vi "route.vi"() -> ()   [LabVIEW 2014]
uses:
  <vilib>/Utility/sysdir.llb/System Directory Type.ctl
  <vilib>/Utility/config.llb/Read Key (String).vi
  <vilib>/Utility/config.llb/Write Key (String).vi
  <vilib>/Utility/config.llb/Read Key (Path).vi
  <vilib>/Utility/config.llb/Write Key (Path).vi
  subVI/departure.vi
  subVI/Destination.vi
  <vilib>/Utility/file.llb/Write To Spreadsheet File (string).vi
  <vilib>/httpClient/LabVIEWHTTPClient.lvlib
  <vilib>/Utility/config.llb/NI_LVConfig.lvlib
panel:
  in  "?":bool
  in  "?":bool
  in  "?":bool
  out "PMDG":string
  out "FS2004/FS9":string
  out "FSX":string
  out "활주로 2":string[](array[string])
  out "초":i32[](array[numeric])
  out "분":i32[](array[numeric])
  out "시":i32[](array[numeric])
  in  "기록":bool
  out "시간 2":string
  in  "확인 버튼 2":bool
  in  "초기화 2":bool
  out "시간":string
  in  "ATC":bool
  out "활주로":string[](array[string])
  out "fms":string
  out "time/시간":dbl
  in  "도움말":bool
  in  "피드백":bool
  in  "저장 경로":path
  out "Distance":string="0"
  in  "찾기":bool
  in  "?":bool
  in  "?":bool
  out "x fmc 플랜":string
  out "FMS 플랜":string
  in  "Destination":string
  in  "departure":string
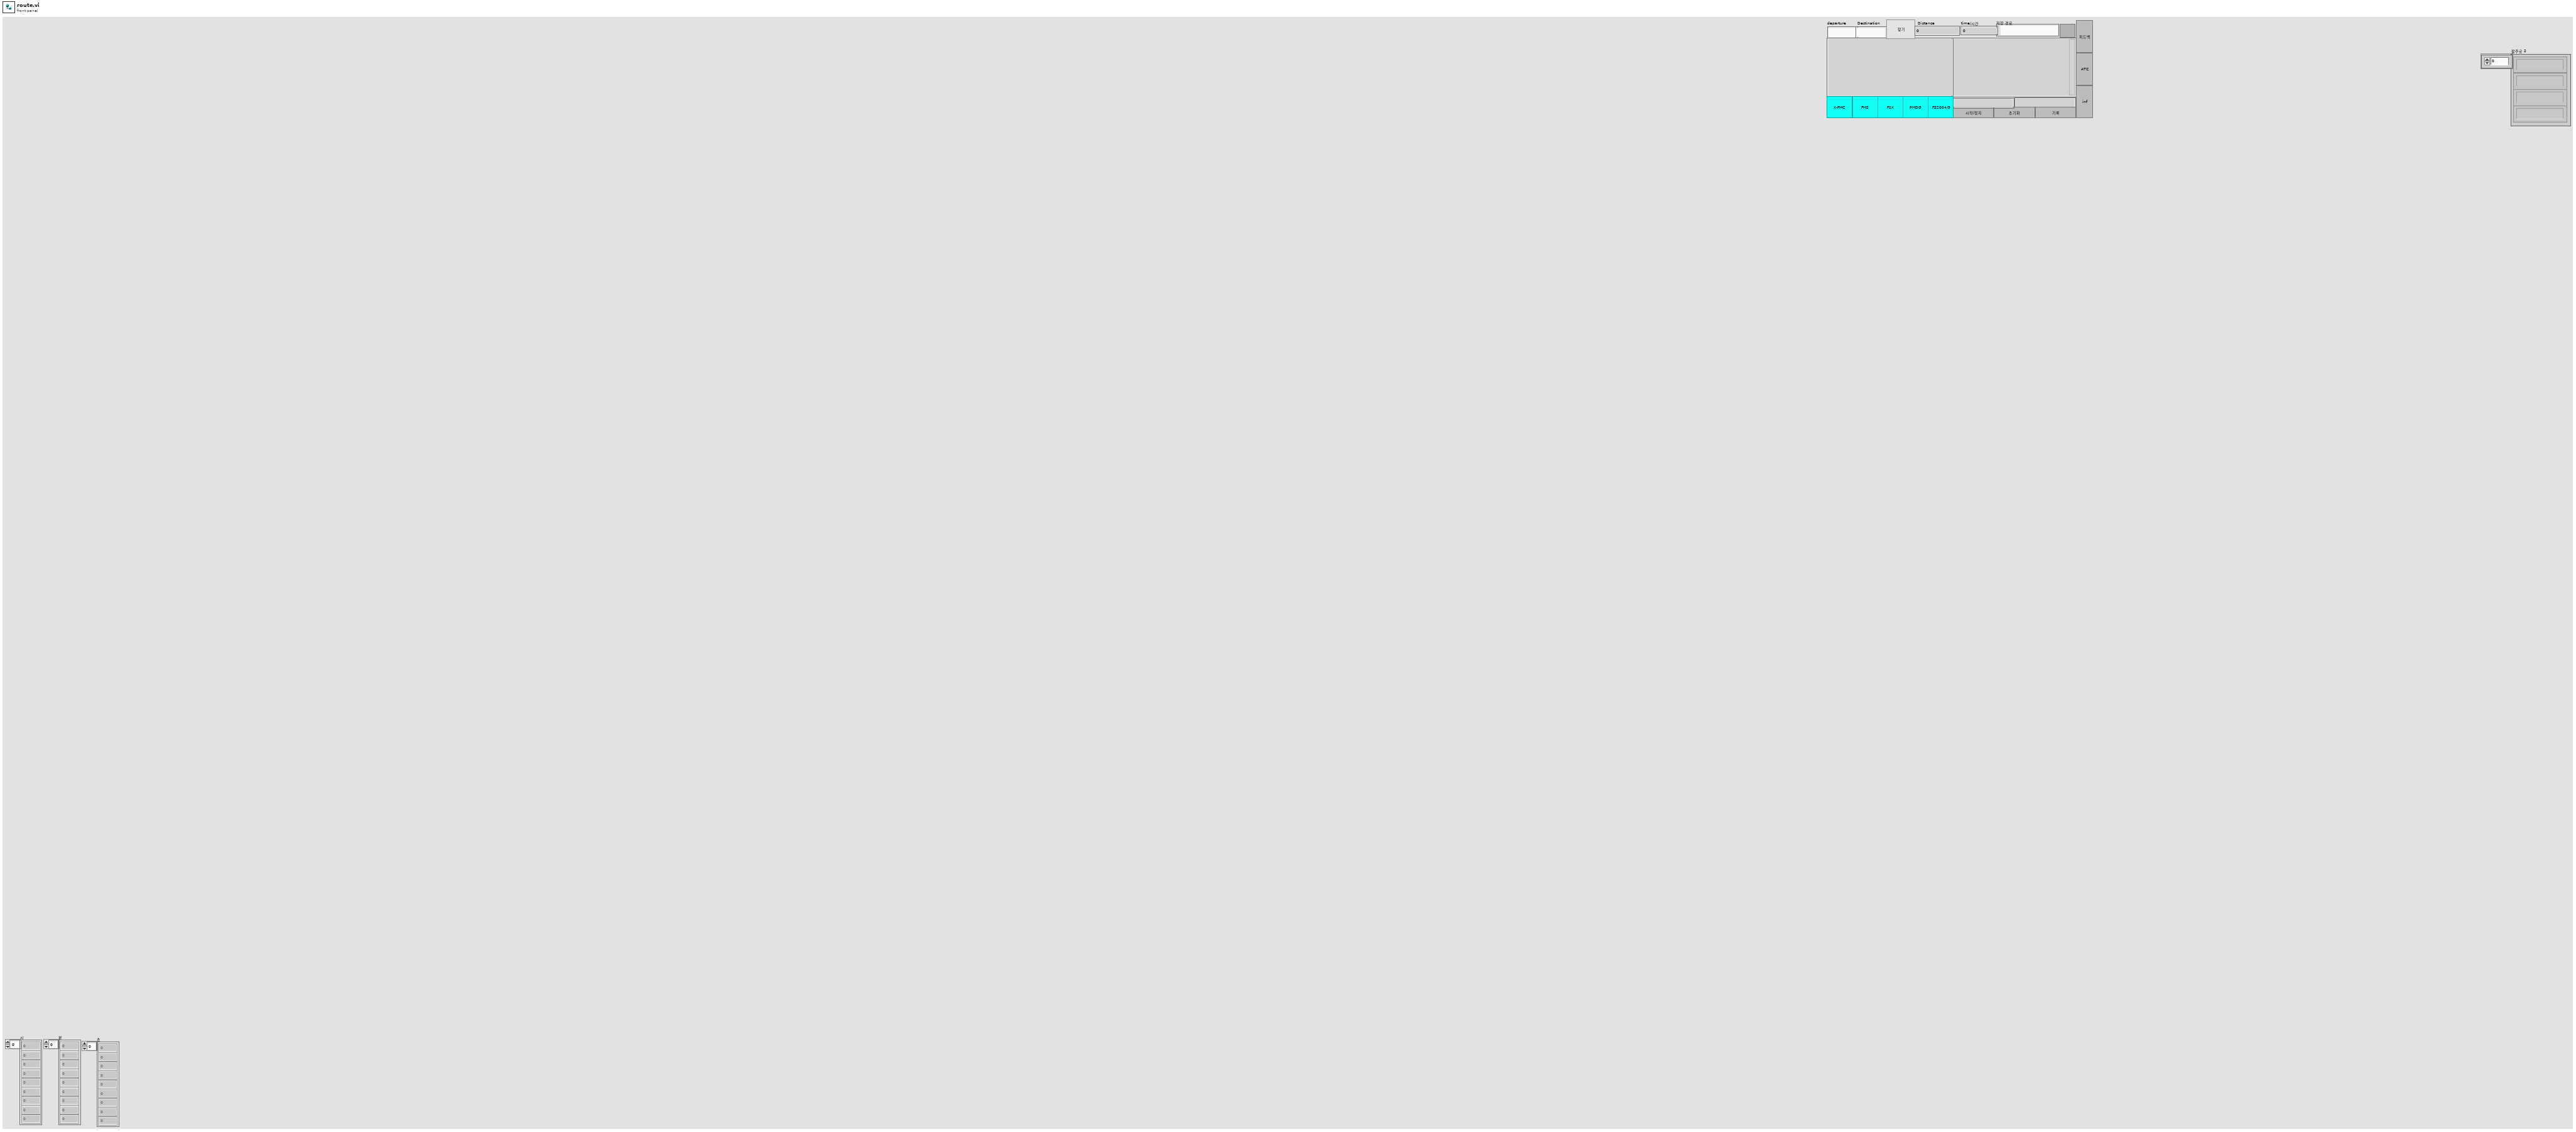
[diagram p1: front panel]
types:
  T1 = enum16{"open", "replace", "create", "open or create", "replace or create", "replace or create with confirmation"}
  T2 = typedef "NI_LVConfig.lvlib/Config Data RefNum.ctl" = refnum<k1>
  T3 = typedef "System Directory Type.ctl" = i32
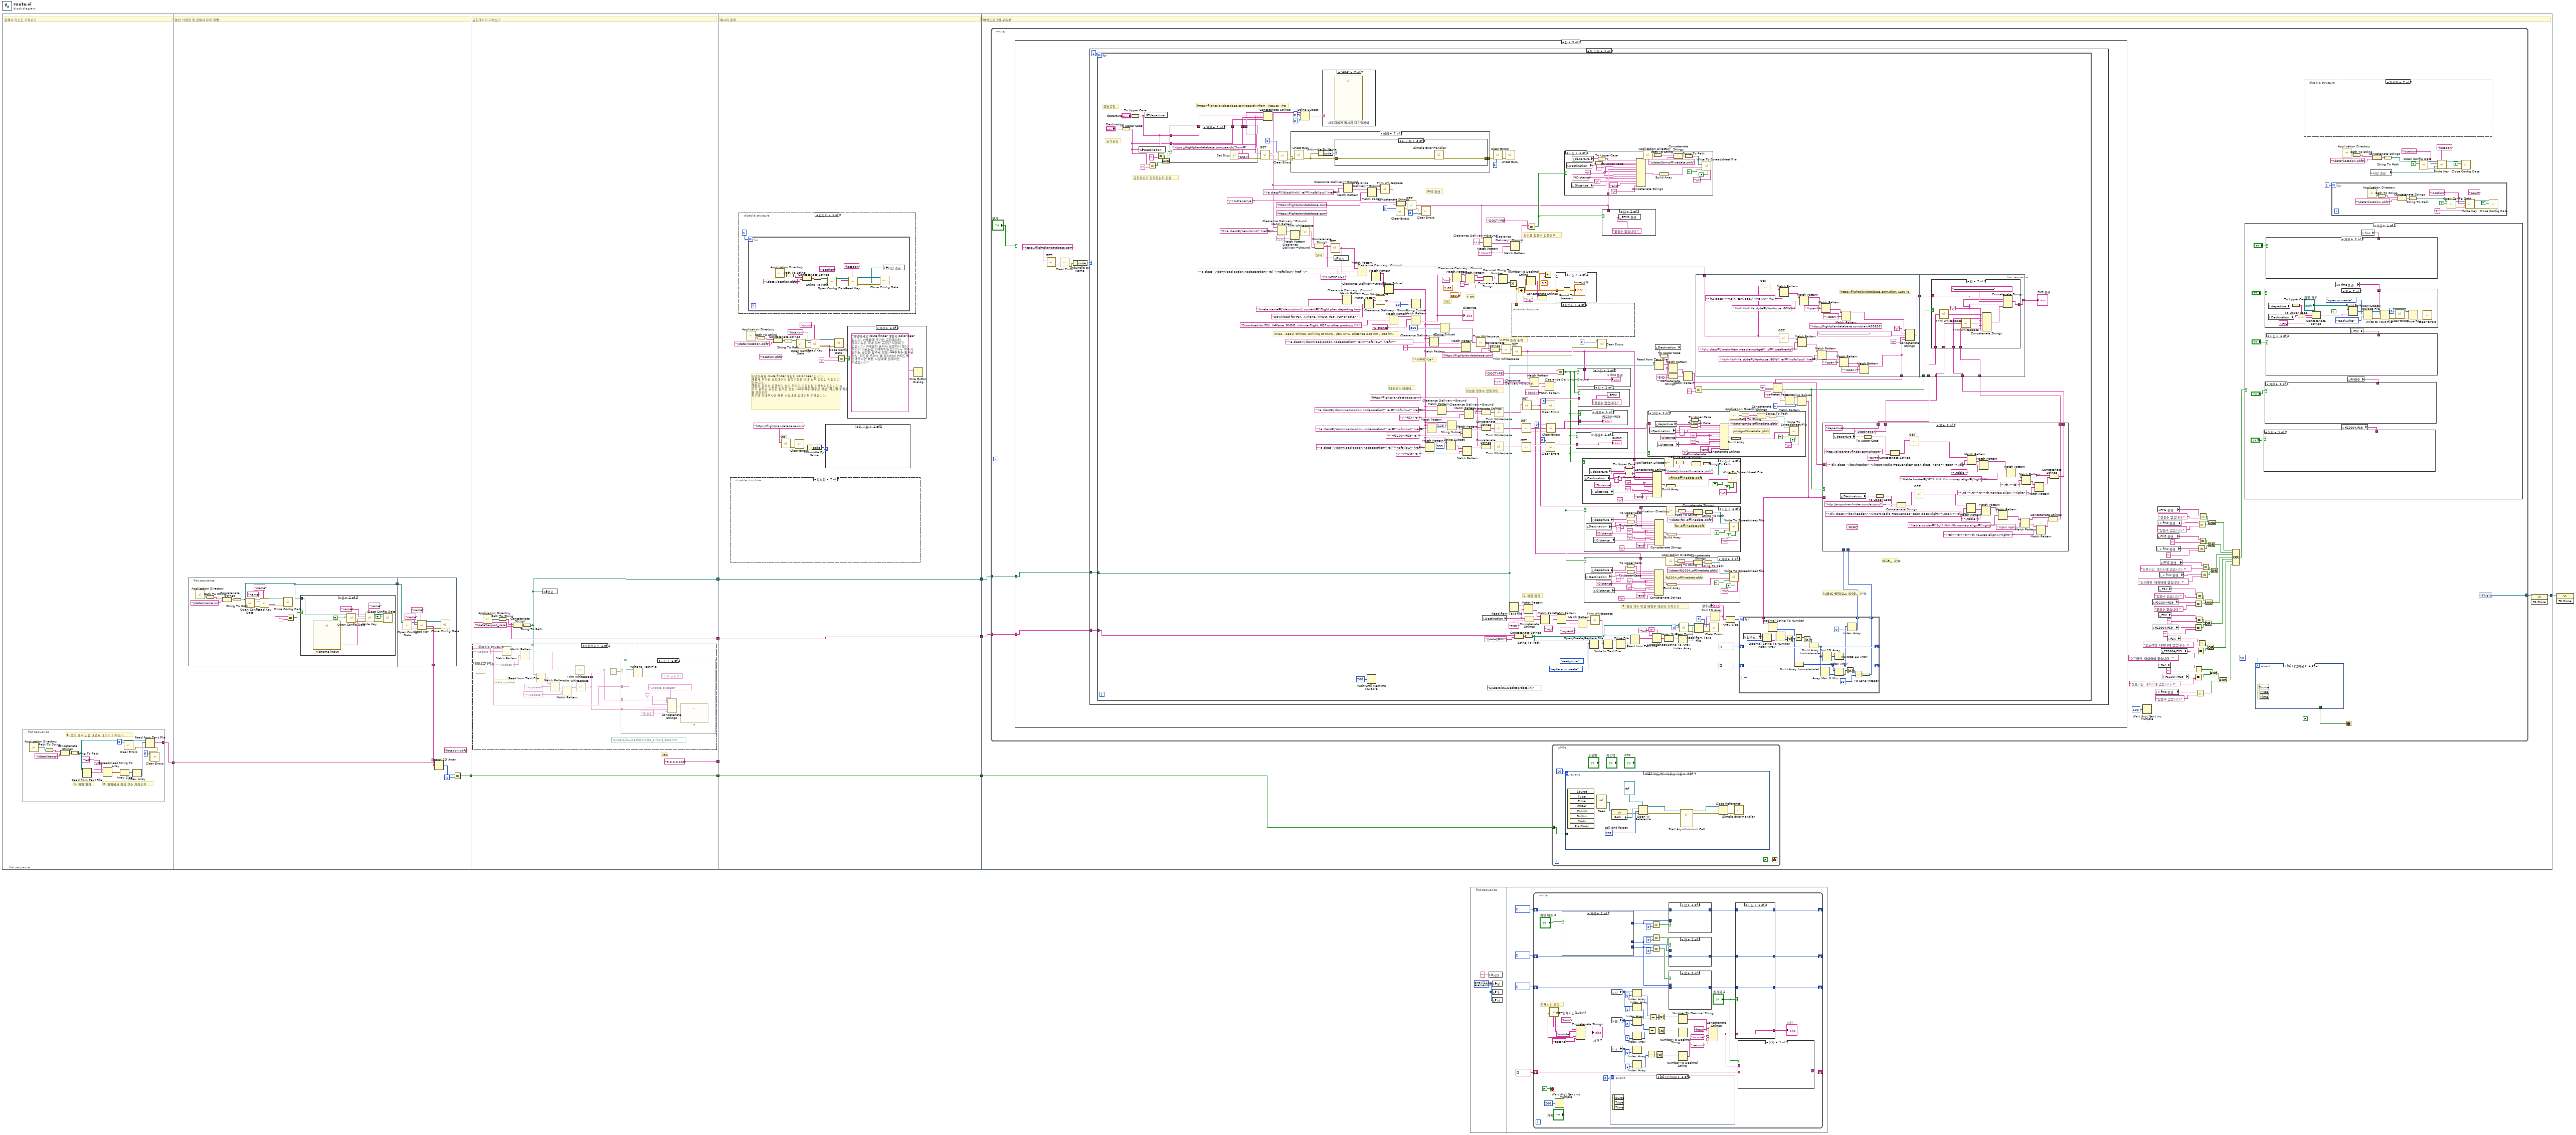
[diagram p0: block diagram]
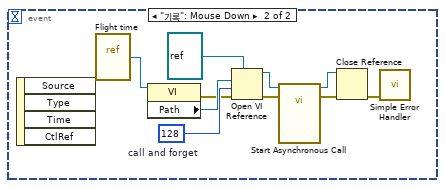
[diagram p2: hidden frame]
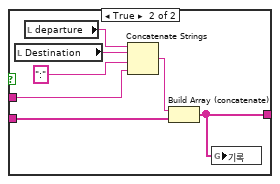
[diagram p3: hidden frame]
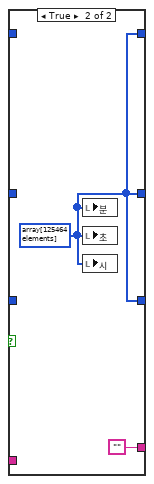
[diagram p4: hidden frame]
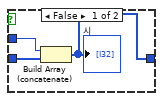
[diagram p5: hidden frame]
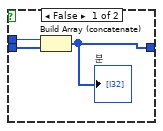
[diagram p6: hidden frame]
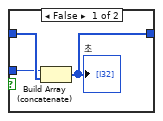
[diagram p7: hidden frame]
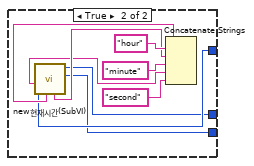
[diagram p8: hidden frame]
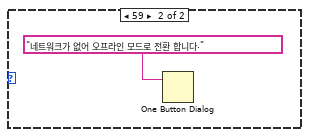
[diagram p13: hidden frame]
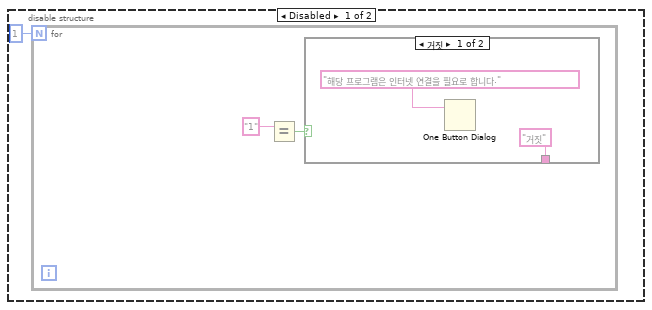
[diagram p14: hidden frame]
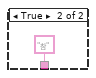
[diagram p15: hidden frame]
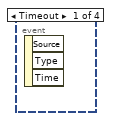
[diagram p17: hidden frame]
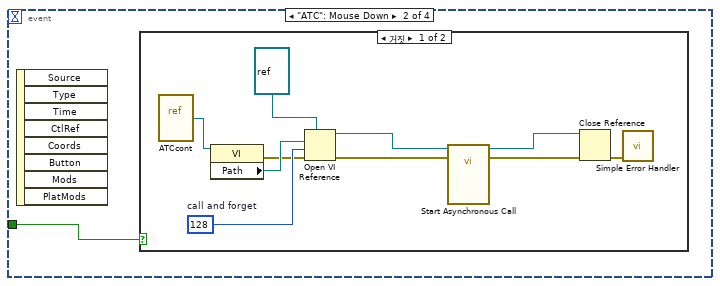
[diagram p18: hidden frame]
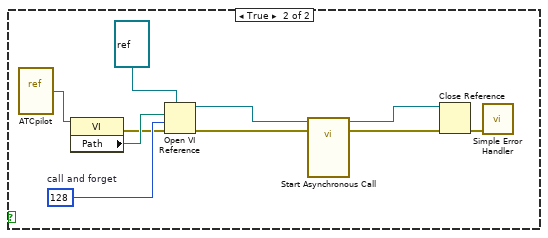
[diagram p19: hidden frame]
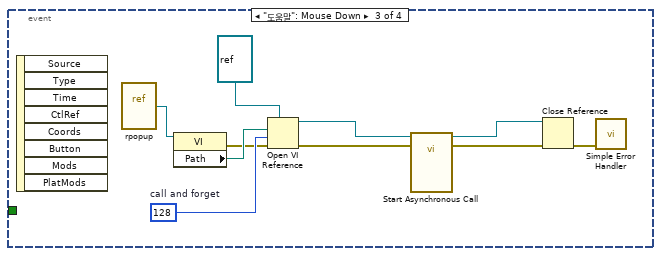
[diagram p20: hidden frame]
diagram:
  n1 = flat-sequence {
    tunnel: [w11] -> w5
    tunnel: w5 -> [w33]
    tunnel: [w31] -> w4
    tunnel: [w69] -> w8
    tunnel: [w70] -> w7
    tunnel: ["3.0.0.0.100"] -> w6
    tunnel: w4 -> [w66]
    tunnel: [w66] -> w3
    tunnel: [w97] -> w10
    tunnel: [w98] -> w9
    tunnel: w8 -> [w97]
    tunnel: w7 -> [w98]
    tunnel: w6 -> [_]
    tunnel: w3 -> [w96]
    tunnel: [w96] -> w2
    tunnel: w10 -> [w142]
    tunnel: w9 -> [w141]
    tunnel: w2 -> [w140]
    tunnel: [w138] -> w1
    frame #0 {
      # "관제사 리스드 가져오기"
      n2 = flat-sequence {
        tunnel: [w16] -> w11
        frame #0 {
          # "3. 행의 갯수 만큼 배열로 데이터 가져오기"
          # "2. 파일에서 행의 갯수 가져오기"
          # "1. 파일 읽기"
          n3 = call <vilib>:"Application Directory.vi"() -> ("Application Directory"=w20:path)
          n4 = Path To String(path=w20) -> (string=w19:string)
          n5 = Concatenate Strings(w19, "\\data\\temp" ("문자열")) -> (w18:string)
          n6 = String To Path(string=w18) -> (path=w17:path)
          n7 = Read from Text File(file (use dialog)=w17) -> (text=w23:string)  [unwired: 1 in, 5 out]
          n8 = Spreadsheet String To Array(delimiter (Tab)="\r", format string="%d", spreadsheet string=w23) -> (array=w25:dbl[][])  [unwired: 1 out]
          n9 = Array Size(array=w25) -> (size(s)=w24:i32[])
          n10 = call <vilib>:"Clear Errors.vi"("specific error code to clear (0: all)"=0) -> ("error out"=w15:errorcluster)  [unwired: 5 in, 1 out]
          n11 = Index Array(array=w24) -> (element=w22:i32)  [unwired: 1 in]
          n12 = Read from Text File(file (use dialog)=w17, count=w22, error in=w15) -> (text=w16:string[], error out=w13:errorcluster)  [unwired: 3 out]
          n13 = call <vilib>:"Clear Errors.vi"("error in (no error)"=w13, "specific error code to clear (0: all)"=0) -> ()  [unwired: 4 in, 2 out]
        }
      }
    }
    frame #1 {
      (unwired) "location.pbfs" ("문자열")
      # "본인 닉네임 및 관제사 유무 판별"
      n14 = flat-sequence {
        tunnel: [w34] -> w28
        tunnel: [w59] -> w30
        tunnel: w28 -> [w58]
        frame #0 {
          n15 = call <vilib>:"Application Directory.vi"() -> ("Application Directory"=w40:path)
          n16 = Path To String(path=w40) -> (string=w38:string)
          n17 = Concatenate Strings(w38, "\\data\\name.ini" ("문자열")) -> (w39:string)
          n18 = String To Path(string=w39) -> (path=w34:path)
          n19 = call <vilib>:"Open Config Data.vi"("configuration file path"=w34) -> ("error out"=w45:errorcluster, "refnum"=w46:T2)  [unwired: 8 in, 1 out]
          n20 = call-poly <vilib>:"Read Key.vi"("section"="name", "error in (no error)"=w45, "key"="name", "refnum"=w46) -> ("error out"=w44:errorcluster, "value"=w35:string, "refnum out"=w43:T2)  [unwired: 4 in, 1 out]
          n21 = call <vilib>:"Close Config Data.vi"("error in (no error)"=w44, "refnum"=w43) -> ()  [unwired: 8 in, 2 out]
          n22 = Equal?(x=w35, y="") -> (x = y?=w36:bool)
          n23 = case shown="참" w36 {
            tunnel: w34 -> [_ w48]
            frame False {
            }
            frame True {
              n24 = call "nicname input"() -> ("nicname"=w49:string)  [unwired: 17 in, 2 out]
              n25 = call <vilib>:"Open Config Data.vi"("create file if necessary (T)"=TRUE, "configuration file path"=w48) -> ("error out"=w51:errorcluster, "refnum"=w52:T2)  [unwired: 7 in, 1 out]
              n26 = call-poly <vilib>:"Write Key.vi"("section"="name", "error in (no error)"=w51, "value"=w49, "key"="name", "refnum"=w52) -> ("error out"=w54:errorcluster, "refnum out"=w53:T2)  [unwired: 4 in, 1 out]
              n27 = call <vilib>:"Close Config Data.vi"("error in (no error)"=w54, "write file if changed (T)"=TRUE, "refnum"=w53) -> ()  [unwired: 7 in, 2 out]
            }
          }
        }
        frame #1 {
          n28 = call <vilib>:"Open Config Data.vi"("configuration file path"=w58) -> ("error out"=w62:errorcluster, "refnum"=w61:T2)  [unwired: 8 in, 1 out]
          n29 = call-poly <vilib>:"Read Key.vi"("section"="name", "error in (no error)"=w62, "key"="name", "refnum"=w61) -> ("error out"=w63:errorcluster, "value"=w59:string, "refnum out"=w64:T2)  [unwired: 4 in, 1 out]
          n30 = call <vilib>:"Close Config Data.vi"("error in (no error)"=w63, "refnum"=w64) -> ()  [unwired: 8 in, 2 out]
        }
      }
      n31 = Search 1D Array(1D array=w33, element=w30) -> (index of element=w32:i32)  [unwired: 1 in]
      n32 = Equal?(x=w32, y=-1) -> (x = y?=w31:bool)
    }
    frame #2 {
      # "VER"
      # "공항데이터 가져오기"
      n33 = call <vilib>:"Application Directory.vi"() -> ("Application Directory"=w72:path)
      n34 = Path To String(path=w72) -> (string=w70:string)
      n35 = Concatenate Strings(w70, "\\data\\airport_data" ("문자열")) -> (w68:string)
      n36 = String To Path(string=w68) -> (path=w69:path)
      n37 = disable-structure shown="비활성화" {
        disable-tunnel: w69 -> [w86 _]
        frame Disabled {
          (unwired) path "C:/Users/lsw/Desktop/KOR_airport_data.txt" ("File Path Control")
          # "data update"
          n38 = call "데이터업데이트.vi"() -> ("data"=w76:string)  [unwired: 11 in]
          n39 = Match Pattern(string=w76, regular expression="<update>" ("정규식")) -> (after substring=w84:string)  [unwired: 1 in, 3 out]
          n40 = Match Pattern(string=w84, regular expression="</update>" ("정규식")) -> (before substring=w78:string)  [unwired: 1 in, 3 out]
          n41 = Read from Text File(file (use dialog)=w86) -> (text=w79:string)  [unwired: 3 in, 3 out]
          n42 = Match Pattern(string=w79, regular expression="<update>" ("정규식")) -> (after substring=w81:string)  [unwired: 1 in, 3 out]
          n43 = Match Pattern(string=w81, regular expression="</update>" ("정규식")) -> (before substring=w77:string)  [unwired: 1 in, 3 out]
          n44 = call <vilib>:"Trim Whitespace.vi"("string"=w78) -> ("trimmed string"=w74:string)  [unwired: 1 in]
          n45 = call <vilib>:"Trim Whitespace.vi"("string"=w77) -> ("trimmed string"=w75:string)  [unwired: 1 in]
          n46 = Equal?(x=w74, y=w75) -> (x = y?=w73:bool)
          n47 = case shown="거짓" w73 {
            tunnel: w86 -> [w95 _]
            tunnel: w76 -> [w89 _]
            tunnel: w75 -> [w88 _]
            tunnel: w74 -> [w87 _]
            frame False {
              n48 = Write to Text File(file (use dialog)=w95, text=w89) -> ()  [unwired: 2 in, 3 out]
              n49 = Concatenate Strings(w87, "update success" ("문자열"), "\r", "기존 버전은", w88, "입니다." ("문자열")) -> (w90:string)
              n50 = call "?"("Message"=w90) -> ()  [unwired: 9 in, 2 out]
            }
            frame True {
            }
          }
        }
        frame Enabled {
        }
      }
      n51 = global write "airport경로.vi" "경로"(w69) -> ()
    }
    frame #3 {
      (unwired) "location.pbfs" ("문자열")
      # "안녕하세요 route finder 개발자 polor bear 입니다. \n새롭게 추가된 공항데이터 출력기능은 국내 일부 공항만 지원되고 있습니다. \n개발자 혼자서 진행하다 보니 무리가 따르는점 이해부탁드립니다.ㅠ \n추가 원하는 공항은 활주로 정보,.ILS주파수,활주로 정보  파드별 주파수 를 정리하여 \n피드백 보내주시면 빠른 시일내에 업데이트 하겟습니다."
      # "메시지 출력"
      n52 = disable-structure shown="활성화" {
        frame Disabled {
          n53 = for {
            N: 1 -> [_]
            n54 = Equal?(x="1" ("y")) -> (x = y?=w121:bool)  [unwired: 1 in]
            n55 = case shown="거짓" w121 {
              tunnel: ["거짓" "참"] -> _
              frame False {
                n56 = One Button Dialog(message="해당 프로그램은 인터넷 연결을 필요로 합니다." ("메시지")) -> ()  [unwired: 1 in, 1 out]
              }
              frame True {
              }
            }
          }
        }
        frame Enabled {
        }
      }
      n57 = disable-structure shown="활성화" {
        frame Enabled {
          n58 = for {
            N: 1 -> [_]
            n59 = call <vilib>:"Application Directory.vi"() -> ("Application Directory"=w129:path)
            n60 = Path To String(path=w129) -> (string=w127:string)
            n61 = Concatenate Strings(w127, "\\data\\location.pbfs" ("문자열")) -> (w128:string)
            n62 = String To Path(string=w128) -> (path=w126:path)
            n63 = call <vilib>:"Open Config Data.vi"("configuration file path"=w126) -> ("error out"=w135:errorcluster, "refnum"=w134:T2)  [unwired: 8 in, 1 out]
            n64 = call-poly <vilib>:"Read Key.vi"("section"="location", "error in (no error)"=w135, "key"="location", "refnum"=w134) -> ("error out"=w136:errorcluster, "value"=w131:path, "refnum out"=w137:T2)  [unwired: 4 in, 1 out]
            n65 = call <vilib>:"Close Config Data.vi"("error in (no error)"=w136, "refnum"=w137) -> ()  [unwired: 8 in, 2 out]
            n66 = local write "저장 경로"(w131) -> ()
          }
        }
        frame Disabled {
        }
      }
      n67 = call <vilib>:"Application Directory.vi"() -> ("Application Directory"=w102:path)
      n68 = Path To String(path=w102) -> (string=w100:string)
      n69 = Concatenate Strings(w100, "\\data\\location.pbfs" ("문자열")) -> (w101:string)
      n70 = call <vilib>:"GET.vi"("url"="https://flightplandatabase.com") -> ("error out"=w116:errorcluster)  [unwired: 11 in, 3 out]
      n71 = String To Path(string=w101) -> (path=w99:path)
      n72 = call <vilib>:"Clear Errors.vi"("error in (no error)"=w116) -> ("error out"=w114:errorcluster)  [unwired: 5 in, 1 out]
      n73 = call <vilib>:"Open Config Data.vi"("configuration file path"=w99) -> ("error out"=w110:errorcluster, "refnum"=w111:T2)  [unwired: 8 in, 1 out]
      n74 = Unbundle By Name(w114) -> ("code"=w113:i32)
      n75 = call-poly <vilib>:"Read Key.vi"("section"="count", "error in (no error)"=w110, "key"="location", "refnum"=w111) -> ("error out"=w109:errorcluster, "value"=w104:string, "refnum out"=w108:T2)  [unwired: 4 in, 1 out]
      n76 = case shown="0, 기본" w113 {
        frame 0, Default {
        }
        frame 59 {
          n77 = One Button Dialog(message="네트워크가 없어 오프라인 모드로 전환 합니다." ("메시지")) -> ()  [unwired: 1 in, 1 out]
        }
      }
      n78 = call <vilib>:"Close Config Data.vi"("error in (no error)"=w109, "refnum"=w108) -> ()  [unwired: 8 in, 2 out]
      n79 = Equal?(x=w104, y="1") -> (x = y?=w106:bool)
      n80 = case shown="거짓" w106 {
        frame False {
          n81 = One Button Dialog(message="안녕하세요 route finder 개발자 polor bear 입니다. \n새롭게 추가된 공항데이터 출력기능은 국내 일부 공항만 지원되고 있습니다. \n개발자 혼자서 진행하다 보니 무리가 따르는점 이해부탁드립니다.ㅠ \n추가 원하는 공항은 활주로 정보,.ILS주파수,활주로 정보  파드별 주파수 를 정리하여 \n피드백 보내주시면 빠른 시일내에 업데이트 하겟습니다." ("메시지")) -> ()  [unwired: 1 in, 1 out]
        }
        frame True {
        }
      }
    }
    frame #4 {
      # "메인프로그램 구동부"
      n82 = while {
        tunnel: w142 -> [w231]
        tunnel: w141 -> [w230]
        tunnel: [w220] -> w139
        stop <- w221 stop-if-true
        (unwired) FALSE
        n83 = case shown="참" "찾기" {
          tunnel: w231 -> [w280 w526]
          tunnel: w230 -> [w279 w525]
          frame False {
            n84 = disable-structure shown="비활성화" {
              disable-tunnel: w280 -> [w282 _]
              disable-tunnel: w279 -> [w281 _]
              frame Disabled {
                n85 = while {
                  tunnel: w282 -> [w297]
                  tunnel: w281 -> [w296]
                  stop <- FALSE stop-if-true
                  (unwired) path "C:/Users/lsw/Desktop/data.ini" ("File Path Control")
                  # "¼Œ·tÇ ÆÅDÇLµ \\ÖüÈ\\¸  ÁÝÐ"
                  # "1. 파일 읽기"
                  # "3. 행의 갯수 만큼 배열로 데이터 가져오기"
                  n86 = local read "Destination"() -> (w284:string)
                  n87 = Wait Until Next ms Multiple(millisecond multiple=u32 1800000 ("ms 배수")) -> ()  [unwired: 1 out]
                  n88 = Equal?(x="", y=w284) -> (x = y?=w285:bool)
                  n89 = case shown="참" w285 {
                    tunnel: w284 -> [_ w355]
                    tunnel: [_ w354] -> w286
                    frame False {
                    }
                    frame True {
                      n90 = To Upper Case(1:w355) -> (0:w354:string)
                    }
                  }
                  n91 = local read "Destination"() -> (w288:string)
                  n92 = Concatenate Strings(w296, "\\data\\RWY" ("문자열")) -> (w350:string)
                  n93 = Read from Text File(file (use dialog)=w297) -> (text=w337:string)  [unwired: 1 in, 5 out]
                  n94 = String To Path(string=w350) -> (path=w352:path)
                  n95 = Equal?(x=w288, y="") -> (x = y?=w289:bool)
                  n96 = Match Pattern(string=w337, regular expression=w286) -> (after substring=w336:string)  [unwired: 1 in, 3 out]
                  n97 = Concatenate Strings(w286, "END;" ("정규식")) -> (w339:string)
                  n98 = case shown="거짓" w289 {
                    tunnel: w288 -> [w356 _]
                    tunnel: [w356 _] -> w290
                    frame False {
                    }
                    frame True {
                    }
                  }
                  n99 = Match Pattern(string=w336, regular expression=w339) -> (before substring=w338:string)  [unwired: 1 in, 3 out]
                  n100 = Match Pattern(string=w338, regular expression="rwy" ("문자열")) -> (after substring=w341:string)  [unwired: 1 in, 3 out]
                  n101 = Read from Text File(file (use dialog)=w297) -> (text=w312:string)  [unwired: 1 in, 5 out]
                  n102 = To Upper Case(1:w290) -> (0:w317:string)
                  n103 = Match Pattern(string=w341, regular expression="rwyand;" ("정규식")) -> (before substring=w342:string)  [unwired: 1 in, 3 out]
                  n104 = Concatenate Strings(w317, "END;" ("정규식")) -> (w314:string)
                  n105 = Match Pattern(string=w312, regular expression=w317) -> (after substring=w316:string)  [unwired: 1 in, 3 out]
                  n106 = call <vilib>:"Trim Whitespace.vi"("string"=w342) -> ("trimmed string"=w343:string)  [unwired: 1 in]
                  n107 = Match Pattern(string=w316, regular expression=w314) -> (before substring=w299:string)  [unwired: 1 in, 3 out]
                  n108 = Open/Create/Replace File(file path (use dialog)=w352, operation (0:open)=T1."replace or create" ("동작(0:open)"), access (0:read/write)=enum16{"read/write", "read-only", "write-only"}."read/write" ("접근(0:읽기/쓰기)")) -> (refnum out=w347:refnum<file>, error out=w344:errorcluster)  [unwired: 3 in, 1 out]
                  n109 = Write to Text File(file (use dialog)=w347, text=w343, error in=w344) -> (refnum out=w346:refnum<file>, error out=w345:errorcluster)  [unwired: 1 in, 1 out]
                  n110 = Equal?(x=w299, y="") -> (x = y?=w298:bool)
                  n111 = Close File(refnum=w346, error in=w345) -> (error out=w318:errorcluster)  [unwired: 1 out]
                  n112 = global read "날시.vi" "날시"() -> (w294:string)
                  n113 = Read from Text File(file (use dialog)=w352, error in=w318) -> (text=w324:string)  [unwired: 5 out]
                  n114 = Spreadsheet String To Array(delimiter (Tab)="\r", format string="%d", spreadsheet string=w324) -> (array=w326:dbl[][])  [unwired: 1 out]
                  n115 = flat-sequence {
                    tunnel: w294 -> [w359]
                    tunnel: [w358] -> w353
                    tunnel: [w357] -> w295
                    tunnel: w301 -> [w386]
                    tunnel: w300 -> [w384]
                    tunnel: w353 -> [w385]
                    tunnel: w303 -> [w383]
                    tunnel: w302 -> [w381]
                    tunnel: [w382] -> w293
                    tunnel: [w380] -> _
                    tunnel: w298 -> [w380]
                    frame #0 {
                      (unwired) "https://flightplandatabase.com/plan/435659"
                      # "https://flightplandatabase.com/plan/425078"
                      n116 = call <vilib>:"GET.vi"("url"=w359) -> ("body"=w379:string)  [unwired: 11 in, 3 out]
                      n117 = call <vilib>:"GET.vi"("url"=w359) -> ("body"=w364:string)  [unwired: 11 in, 3 out]
                      n118 = Match Pattern(string=w379, regular expression="<h2 class=\"main-item-title\">METAR</h2>" ("정규식")) -> (after substring=w377:string)  [unwired: 1 in, 3 out]
                      n119 = Match Pattern(string=w364, regular expression="<div class=\"main-item weather-widget\" id=\"weather-to\">" ("정규식")) -> (after substring=w366:string)  [unwired: 1 in, 3 out]
                      n120 = Match Pattern(string=w377, regular expression="<br><br><a style=\"font-size: 80%\" " ("정규식")) -> (before substring=w375:string)  [unwired: 1 in, 3 out]
                      n121 = Match Pattern(string=w366, regular expression="<br><br><a style=\"font-size: 80%\" rel=\"nofollow\" href=\"" ("정규식")) -> (before substring=w368:string)  [unwired: 1 in, 3 out]
                      n122 = Match Pattern(string=w375, regular expression="<span>" ("정규식")) -> (after substring=w373:string)  [unwired: 1 in, 3 out]
                      n123 = Match Pattern(string=w368, regular expression="<span>" ("정규식")) -> (after substring=w370:string)  [unwired: 1 in, 3 out]
                      n124 = Match Pattern(string=w373, regular expression="</span>" ("정규식")) -> (before substring=w361:string)  [unwired: 1 in, 3 out]
                      n125 = Match Pattern(string=w370, regular expression="</span>" ("정규식")) -> (before substring=w357:string)  [unwired: 1 in, 3 out]
                      n126 = Concatenate Strings(w361, "\r", "-------------------------------------------------" ("문자열"), "\r", w357) -> (w358:string)
                    }
                    frame #1 {
                      n127 = case shown="참" w380 {
                        tunnel: w386 -> [w394 w404]
                        tunnel: w385 -> [w395 w403]
                        tunnel: w384 -> [w387 w402]
                        tunnel: w383 -> [_ w400]
                        tunnel: w381 -> [w390 w398]
                        tunnel: [w393 w397] -> w382
                        frame False {
                          w389 = "\r"
                          n128 = call <vilib>:"Trim Whitespace.vi"("string"=w387) -> ("trimmed string"=w388:string)  [unwired: 1 in]
                          n129 = Concatenate Strings(w390, w389, w389, w394, w389, w388) -> (w391:string)
                          n130 = call <vilib>:"Trim Whitespace.vi"("string"=w391) -> ("trimmed string"=w392:string)  [unwired: 1 in]
                          n131 = Concatenate Strings(w395, w389, "--------------frequency------------" ("문자열"), w389, w392) -> (w393:string)
                        }
                        frame True {
                          w405 = "\r"
                          n132 = call <vilib>:"Trim Whitespace.vi"("string"=w400) -> ("trimmed string"=w401:string)  [unwired: 1 in]
                          n133 = call <vilib>:"Trim Whitespace.vi"("string"=w398) -> ("trimmed string"=w399:string)  [unwired: 1 in]
                          n134 = Concatenate Strings(w401, w405, w404, w405, w399, w405, w402, w405) -> (w406:string)
                          n135 = Concatenate Strings(w403, w405, "----------------------------------------" ("문자열"), w405, w406) -> (w397:string)
                        }
                      }
                    }
                  }
                  n136 = Array Size(array=w326) -> (size(s)=w325:i32[])
                  n137 = Index Array(array=w325) -> (element=w323:i32)  [unwired: 1 in]
                  n138 = call <vilib>:"Clear Errors.vi"("specific error code to clear (0: all)"=0) -> ("error out"=w329:errorcluster)  [unwired: 5 in, 1 out]
                  n139 = Read from Text File(file (use dialog)=w352, count=w323, error in=w329) -> (text=w333:string[], error out=w331:errorcluster)  [unwired: 3 out]
                  n140 = call <vilib>:"Clear Errors.vi"("error in (no error)"=w331, "specific error code to clear (0: all)"=0) -> ()  [unwired: 4 in, 2 out]
                  n141 = Match Pattern(string=w295, regular expression="Z" ("정규식")) -> (after substring=w308:string)  [unwired: 1 in, 3 out]
                  n142 = Sort 1D Array(array=w333) -> (sorted array=w319:string[])
                  "활주로 2" <- w319
                  n143 = Match Pattern(string=w308, regular expression="KT" ("정규식")) -> (before substring=w310:string)  [unwired: 1 in, 3 out]
                  n144 = Array Size(array=w319) -> (size(s)=w321:i32)
                  n145 = String Subset(string=w310, length (rest)=4 ("길이(나머지)")) -> (substring=w306:string)  [unwired: 1 in]
                  n146 = for {
                    N: w321 -> [_]
                    shift-right: [w519] -> _
                    shift-left: i32[] [] -> [w523]
                    shift-right: [w505] -> _
                    shift-left: i32[] [] -> [w517]
                    tunnel: w306 -> [w509]
                    tunnel: [w506] -> w304 mode=indexing
                    tunnel: [w503] -> w305 mode=indexing
                    i -> [w524]
                    n147 = local read "활주로 2"() -> (w522:string[])
                    n148 = Index Array(array=w522, index=w524) -> (element=w521:string)
                    n149 = Decimal String To Number(string=w521) -> (number=w513:i32)  [unwired: 2 in, 1 out]
                    n150 = Decimal String To Number(string=w509) -> (number=w508:i32)  [unwired: 2 in, 1 out]
                    n151 = Absolute Value(x=w513) -> (abs(x)=w507:i32)
                    n152 = Subtract(x=w508, y=w507) -> (x-y=w512:i32)
                    n153 = Build Array (concatenate)(w507, w517) -> (w505:i32[])
                    n154 = Absolute Value(x=w512) -> (abs(x)=w511:i32)
                    n155 = Build Array (concatenate)(w511, w523) -> (w519:i32[])
                    n156 = Array Max & Min(array=w519) -> (min index (indices)=w518:i32)  [unwired: 3 out]
                    n157 = Sort 1D Array(array=w519) -> (sorted array=w520:i32[])
                    n158 = Reverse 1D Array(array=w520) -> ()  [unwired: 1 out]
                    n159 = Index Array(array=w505, index=w518) -> (element=w514:i32)
                    n160 = Absolute Value(x=w514) -> (abs(x)=w515:i32)
                    n161 = Index Array(array=w505, index=0 ("인덱스")) -> (element=w503:i32)
                    n162 = Divide(x=w515, y=10) -> (x/y=w510:dbl)
                    n163 = To Long Integer(number=w510) -> (32bit integer=w506:i32)
                  }
                  n164 = case shown="거짓" w298 {
                    tunnel: [_ w470] -> w301
                    tunnel: [w413 w469] -> w300
                    tunnel: w299 -> [w414 _]
                    tunnel: [_ "departure"] -> w303
                    tunnel: [_ " Destination"] -> w302
                    tunnel: w304 -> [w412 _]
                    tunnel: w306 -> [w410 _]
                    tunnel: w305 -> [w408 _]
                    frame False {
                      n165 = Equal?(x=w410, y="") -> (x = y?=w411:bool)
                      n166 = case shown="참" w411 {
                        tunnel: w414 -> [w428 w440]
                        tunnel: [w420 w441] -> w413
                        tunnel: w412 -> [w417 _]
                        tunnel: w408 -> [_ w438]
                        frame False {
                          w423 = "\r"
                          # "õ¬mÕüÈÓÂ œÍ%¸"
                          # "\\ÖüÈ\\¸  ÁÝÐ"
                          n167 = Index Array(array=w417, index=0 ("인덱스")) -> (element=w415:i32)
                          n168 = Number To Decimal String(number=w415) -> (decimal integer string=w429:string)  [unwired: 1 in]
                          n169 = Match Pattern(string=w428, regular expression="frequency") -> (after substring=w433:string)  [unwired: 1 in, 3 out]
                          n170 = Concatenate Strings("frequency", "and;") -> (w432:string)
                          n171 = Concatenate Strings("rwy", w429) -> (w427:string)
                          n172 = Match Pattern(string=w433, regular expression=w432) -> (before substring=w419:string)  [unwired: 1 in, 3 out]
                          n173 = Concatenate Strings(w429, "and") -> (w425:string)
                          n174 = Match Pattern(string=w428, regular expression=w427) -> (after substring=w426:string)  [unwired: 1 in, 3 out]
                          n175 = call <vilib>:"Trim Whitespace.vi"("string"=w419) -> ("trimmed string"=w418:string)  [unwired: 1 in]
                          n176 = Match Pattern(string=w426, regular expression=w425) -> (before substring=w422:string)  [unwired: 1 in, 3 out]
                          n177 = Concatenate Strings(w418, w423, "----------------RWY--------------", w423, w422) -> (w421:string)
                          n178 = call <vilib>:"Trim Whitespace.vi"("string"=w421) -> ("trimmed string"=w420:string)  [unwired: 1 in]
                        }
                        frame True {
                          w446 = "\r"
                          # "õ¬mÕüÈÓÂ œÍ%¸"
                          # "\\ÖüÈ\\¸  ÁÝÐ"
                          n179 = Index Array(array=w438, index=0 ("인덱스")) -> (element=w437:i32)
                          n180 = Number To Decimal String(number=w437) -> (decimal integer string=w451:string)  [unwired: 1 in]
                          n181 = Match Pattern(string=w440, regular expression="frequency") -> (after substring=w455:string)  [unwired: 1 in, 3 out]
                          n182 = Concatenate Strings("frequency", "and;") -> (w454:string)
                          n183 = Concatenate Strings("rwy", w451) -> (w450:string)
                          n184 = Match Pattern(string=w455, regular expression=w454) -> (before substring=w443:string)  [unwired: 1 in, 3 out]
                          n185 = Concatenate Strings(w451, "and") -> (w448:string)
                          n186 = Match Pattern(string=w440, regular expression=w450) -> (after substring=w449:string)  [unwired: 1 in, 3 out]
                          n187 = call <vilib>:"Trim Whitespace.vi"("string"=w443) -> ("trimmed string"=w442:string)  [unwired: 1 in]
                          n188 = Match Pattern(string=w449, regular expression=w448) -> (before substring=w445:string)  [unwired: 1 in, 3 out]
                          n189 = Concatenate Strings(w442, w446, "----------------RWY--------------", w446, w445) -> (w444:string)
                          n190 = call <vilib>:"Trim Whitespace.vi"("string"=w444) -> ("trimmed string"=w441:string)  [unwired: 1 in]
                        }
                      }
                    }
                    frame True {
                      (unwired) "RKPC" ("문자열")
                      (unwired) "RKSS" ("문자열")
                      n191 = local read "Destination"() -> (w460:string)
                      n192 = local read "departure"() -> (w463:string)
                      n193 = Equal?(x="", y=w463) -> (x = y?=w464:bool)
                      n194 = Equal?(x="", y=w460) -> (x = y?=w461:bool)
                      n195 = case shown="참" w464 {
                        tunnel: w463 -> [w502 _]
                        tunnel: [w501 _] -> w466
                        frame False {
                          n196 = To Upper Case(1:w502) -> (0:w501:string)
                        }
                        frame True {
                        }
                      }
                      n197 = case shown="거짓" w461 {
                        tunnel: w460 -> [w500 _]
                        tunnel: [w499 _] -> w465
                        frame False {
                          n198 = To Upper Case(1:w500) -> (0:w499:string)
                        }
                        frame True {
                        }
                      }
                      n199 = Concatenate Strings("http://airportnavfinder.com/airport/", w466) -> (w498:string)
                      n200 = Concatenate Strings("http://airportnavfinder.com/airport/", w465) -> (w472:string)
                      n201 = call <vilib>:"GET.vi"("url"=w472) -> ("body"=w474:string)  [unwired: 11 in, 3 out]
                      n202 = call <vilib>:"GET.vi"("url"=w498) -> ("body"=w496:string)  [unwired: 11 in, 3 out]
                      n203 = Match Pattern(string=w496, regular expression="<div class=\"boxheader\">Airport Radio Frequencies<span class=right></span></div>" ("정규식")) -> (after substring=w494:string)  [unwired: 1 in, 3 out]
                      n204 = Match Pattern(string=w474, regular expression="<div class=\"boxheader\">Airport Radio Frequencies<span class=right></span></div>" ("정규식")) -> (after substring=w476:string)  [unwired: 1 in, 3 out]
                      n205 = Match Pattern(string=w494, regular expression="</table>" ("정규식")) -> (before substring=w492:string)  [unwired: 1 in, 3 out]
                      n206 = Match Pattern(string=w476, regular expression="</table>" ("정규식")) -> (before substring=w471:string)  [unwired: 1 in, 3 out]
                      n207 = Match Pattern(string=w492, regular expression="<table border=\"0\"><tr><th nowrap align=\"right\">" ("정규식")) -> (after substring=w490:string)  [unwired: 1 in, 3 out]
                      n208 = Match Pattern(string=w471, regular expression="<table border=\"0\"><tr><th nowrap align=\"right\">" ("정규식")) -> (after substring=w479:string)  [unwired: 1 in, 3 out]
                      n209 = Match Pattern(string=w490, regular expression="</th><td>" ("정규식")) -> (before substring=w486:string, after substring=w488:string)  [unwired: 1 in, 2 out]
                      n210 = Match Pattern(string=w479, regular expression="</th><td>" ("정규식")) -> (before substring=w483:string, after substring=w481:string)  [unwired: 1 in, 2 out]
                      n211 = Match Pattern(string=w488, regular expression="</td></tr><tr><th nowrap align=\"right\">" ("정규식")) -> (before substring=w485:string)  [unwired: 1 in, 3 out]
                      n212 = Match Pattern(string=w481, regular expression="</td></tr><tr><th nowrap align=\"right\">" ("정규식")) -> (before substring=w484:string)  [unwired: 1 in, 3 out]
                      n213 = Concatenate Strings(w486, w485) -> (w470:string)
                      n214 = Concatenate Strings(w483, w484) -> (w469:string)
                    }
                  }
                  n215 = local write "FMS 플랜"(w293) -> ()
                }
              }
              frame Enabled {
              }
            }
          }
          frame True {
            n216 = call <vilib>:"GET.vi"("url"="https://flightplandatabase.com") -> ("error out"=w530:errorcluster)  [unwired: 11 in, 3 out]
            n217 = call <vilib>:"Clear Errors.vi"("error in (no error)"=w530) -> ("error out"=w528:errorcluster)  [unwired: 5 in, 1 out]
            n218 = Unbundle By Name(w528) -> ("code"=w527:i32)
            n219 = case shown="0, 기본" w527 {
              tunnel: w526 -> [w533 _]
              tunnel: w525 -> [w532 _]
              frame 0, Default {
                n220 = for {
                  N: 1 -> [_]
                  tunnel: w533 -> [w623]
                  tunnel: w532 -> [w633]
                  w575 = "https://flightplandatabase.com" ("url")
                  (unwired) path "C:/Users/lsw/Desktop/data.ini" ("File Path Control")
                  # "다운로드 데이터"
                  # "¼Œ·tÇ ÆÅDÇLµ \\ÖüÈ\\¸  ÁÝÐ"
                  # "\\ÖüÈ\\¸  ÁÝÐ"
                  # "1. 파일 읽기"
                  # "3. 행의 갯수 만큼 배열로 데이터 가져오기"
                  # "날시"
                  # "1.85"
                  # "RKSS - Seoul Gimpo, arriving at RKPC - JEJU INTL. Distance 245 nm / 453 km."
                  # "\">X-FMC</a>"
                  # "https://flightplandatabase.com/search/?from=rkss&to=rjtt"
                  # "FMS 플랜"
                  # "거리"
                  # "X-FMC 플랜 출력"
                  # "정보를 찾을수 없을경우"
                  # "정보를 찾을수 없을경우"
                  # "공항정보가 입력됫는지 판별"
                  # "도착공항"
                  # "출발공항"
                  n221 = To Upper Case(1:"Destination") -> (0:w647:string)
                  n222 = To Upper Case(1:"departure") -> (0:w649:string)
                  n223 = global write "Destination.vi" "Destination"(w647) -> ()
                  n224 = global write "departure.vi" "departure"(w649) -> ()
                  n225 = Equal?(x=w647, y="") -> (x = y?=w676:bool)
                  n226 = Equal?(x=w649, y="") -> (x = y?=w675:bool)
                  n227 = And(x=w675, y=w676) -> (x .and. y?=w677:bool)
                  n228 = case shown="거짓" w677 {
                    tunnel: ["&to=" ("문자열") _] -> w671
                    tunnel: ["https://flightplandatabase.com/search/?from=" ("문자열") _] -> w670
                    tunnel: w647 -> [w1015 _]
                    tunnel: [w1015 "" ("Destination")] -> w669
                    tunnel: [w1014 "" ("departure")] -> w668
                    tunnel: w649 -> [w1014 _]
                    frame False {
                    }
                    frame True {
                      n229 = One Button Dialog(message="경로 입력이 안됫습니다." ("메시지")) -> ()  [unwired: 1 in, 1 out]
                    }
                  }
                  n230 = call <vilib>:"Set Busy.vi"() -> ("error out"=w722:errorcluster)  [unwired: 10 in, 1 out]
                  n231 = Concatenate Strings(w670, w668, w671, w669) -> (w654:string)
                  n232 = call <vilib>:"GET.vi"("url"=w654, "error in (no error)"=w722) -> ("headers"=w726:string, "body"=w547:string, "error out"=w686:errorcluster)  [unwired: 10 in, 1 out]
                  n233 = Match Pattern "Clearance Delivery~Ground"(string=w547, regular expression="\t<a class=\"result-link\" href=\"" ("정규식")) -> (after substring=w715:string)  [unwired: 1 in, 3 out]
                  n234 = call <vilib>:"Clear Errors.vi"("error in (no error)"=w686, "specific error code to clear (0: all)"=0) -> ("error out"=w687:errorcluster)  [unwired: 4 in, 1 out]
                  n235 = Match Pattern "Clearance Delivery~Ground"(string=w715, regular expression="\">" ("정규식")) -> (before substring=w712:string)  [unwired: 1 in, 3 out]
                  n236 = case shown="에러" w687 {
                    selector: w687 -> [w1025 w1028]
                    tunnel: [w1025 w1026] -> w683
                    frame No Error {
                    }
                    frame Error {
                      n237 = call <vilib>:"Unset Busy.vi"("error in (no error)"=w1028) -> ("error out"=w1027:errorcluster)  [unwired: 10 in]
                      n238 = Unbundle By Name(w1027) -> ("code"=w1029:i32)
                      n239 = case shown="2, 기본" w1029 {
                        tunnel: w1027 -> [w1030 w1035 w1037]
                        tunnel: [w1030 w1035 w1036] -> w1026
                        frame 59 {
                          n240 = One Button Dialog(message="에러가 발생하였습니다. 종료하려면 확인 버튼을 누르세요" ("메시지")) -> (true=w1031:bool)  [unwired: 1 in]
                          n241 = Stop(stop? (T)=w1031) -> ()
                        }
                        frame 1 {
                          n242 = One Button Dialog(message="루트를 입력하여 주세요. 종료하려면 확인 버튼을 눌러 주세요" ("메시지")) -> (true=w1033:bool)  [unwired: 1 in]
                          n243 = Stop(stop? (T)=w1033) -> ()
                        }
                        frame 2, Default {
                          n244 = call <vilib>:"Simple Error Handler.vi"("error in (no error)"=w1037) -> ("error out"=w1036:errorcluster)  [unwired: 4 in, 4 out]
                        }
                      }
                    }
                  }
                  n245 = String Subset(string=w726, offset (0)=9 ("오프셋(0)"), length (rest)=3 ("길이(나머지)")) -> (substring=w723:string)
                  n246 = call <vilib>:"Trim Whitespace.vi"("string"=w712) -> ("trimmed string"=w710:string)  [unwired: 1 in]
                  n247 = Concatenate Strings("https://flightplandatabase.com" ("url"), w710) -> (w643:string)
                  n248 = case shown="\"404\"" w723 {
                    frame "거짓", Default {
                    }
                    frame "404" {
                      n249 = call "사용자에게 메시지 디스플레이"() -> ()  [unwired: 10 in, 2 out]
                    }
                  }
                  n250 = call <vilib>:"GET.vi"("url"=w643) -> ("body"=w653:string)  [unwired: 11 in, 3 out]
                  n251 = global write "날시.vi" "날시"(w643) -> ()
                  n252 = Match Pattern "Clearance Delivery~Ground"(string=w653, regular expression="<meta name=\"description\" content=\"Flight plan departing from " ("정규식")) -> (after substring=w701:string)  [unwired: 1 in, 3 out]
                  n253 = Match Pattern "Clearance Delivery~Ground"(string=w547, regular expression="<a class=\"block-link\" rel=\"nofollow\" href=\"" ("정규식")) -> (after substring=w720:string)  [unwired: 1 in, 3 out]
                  n254 = Match Pattern "Clearance Delivery~Ground"(string=w653, regular expression="<a class=\"download-option nodecoration\" rel=\"nofollow\" href=\"" ("정규식")) -> (after substring=w581:string)  [unwired: 1 in, 3 out]
                  n255 = Match Pattern "Clearance Delivery~Ground"(string=w701, regular expression="Download for FSX, X-Plane, PMDG, FS9, PDF or other " ("정규식")) -> (before substring=w703:string)  [unwired: 1 in, 3 out]
                  n256 = Wait Until Next ms Multiple(millisecond multiple=u32 200 ("ms 배수")) -> ()  [unwired: 1 out]
                  n257 = Match Pattern "Clearance Delivery~Ground"(string=w720, regular expression="\">X-Plane</a>" ("정규식")) -> (before substring=w718:string)  [unwired: 1 in, 3 out]
                  n258 = Match Pattern "Clearance Delivery~Ground"(string=w581, regular expression="\">X-FMC</a>" ("정규식")) -> (before substring=w707:string)  [unwired: 1 in, 3 out]
                  n259 = call <vilib>:"Trim Whitespace.vi"("string"=w703) -> ("trimmed string"=w551:string)  [unwired: 1 in]
                  n260 = call <vilib>:"Trim Whitespace.vi"("string"=w718) -> ("trimmed string"=w546:string)  [unwired: 1 in]
                  n261 = String Subset(string=w707) -> (substring=w536:string)  [unwired: 2 in]
                  n262 = Match Pattern(string=w551, regular expression="Download for FSX, X-Plane, PMDG, Infinite Flight, PDF or other products.\">" ("정규식")) -> (before substring=w550:string)  [unwired: 1 in, 3 out]
                  n263 = call <vilib>:"Clear Errors.vi"("specific error code to clear (0: all)"=0) -> ("error out"=w568:errorcluster)  [unwired: 5 in, 1 out]
                  n264 = Concatenate Strings("https://flightplandatabase.com" ("url"), w546) -> (w716:string)
                  n265 = call <vilib>:"GET.vi"("url"=w716, "error in (no error)"=w568) -> ("body"=w548:string, "error out"=w566:errorcluster)  [unwired: 10 in, 2 out]
                  n266 = Match Pattern(string=w550, regular expression="Distance" ("정규식")) -> (after substring=w549:string)  [unwired: 1 in, 3 out]
                  "Distance" <- w549
                  n267 = String Subset(string=w551, offset (0)=60 ("오프셋(0)")) -> ()  [unwired: 1 in, 1 out]
                  n268 = call <vilib>:"Clear Errors.vi"("error in (no error)"=w566, "specific error code to clear (0: all)"=0) -> ()  [unwired: 4 in, 2 out]
                  n269 = Match Pattern ("Clearance Delivery~Ground")(string=w536, regular expression="<a class=\"download-option nodecoration\" rel=\"nofollow\" href=\"" ("정규식")) -> ()  [unwired: 1 in, 4 out]
                  n270 = Match Pattern ("Clearance Delivery~Ground")(string=w536, regular expression="<a class=\"download-option nodecoration\" rel=\"nofollow\" href=\"" ("정규식")) -> ()  [unwired: 1 in, 4 out]
                  n271 = Match Pattern "Clearance Delivery~Ground"(string=w536, regular expression="<a class=\"download-option nodecoration\" rel=\"nofollow\" href=\"" ("정규식")) -> (after substring=w543:string)  [unwired: 1 in, 3 out]
                  n272 = Match Pattern "Clearance Delivery~Ground"(string=w536, regular expression="<a class=\"download-option nodecoration\" rel=\"nofollow\" href=\"" ("정규식")) -> (after substring=w580:string)  [unwired: 1 in, 3 out]
                  n273 = String Subset(string=w536, offset (0)=810 ("오프셋(0)")) -> (substring=w542:string)  [unwired: 1 in]
                  n274 = String Subset(string=w536, offset (0)=595 ("오프셋(0)")) -> (substring=w537:string)  [unwired: 1 in]
                  n275 = String Subset(string=w536, offset (0)=225 ("오프셋(0)")) -> (substring=w538:string)  [unwired: 1 in]
                  n276 = Match Pattern "Clearance Delivery~Ground"(string=w549, regular expression="nm" ("정규식")) -> (before substring=w664:string)  [unwired: 1 in, 3 out]
                  n277 = Match Pattern ("Clearance Delivery~Ground")(string=w543, regular expression="" ("정규식")) -> ()  [unwired: 1 in, 4 out]
                  n278 = Match Pattern ("Clearance Delivery~Ground")(string=w538, regular expression="\">FS2004/FS9</a>" ("정규식")) -> (before substring=w578:string)  [unwired: 1 in, 3 out]
                  n279 = Match Pattern ("Clearance Delivery~Ground")(string=w537, regular expression="\">PMDG</a>" ("정규식")) -> (before substring=w574:string)  [unwired: 1 in, 3 out]
                  n280 = Match Pattern "Clearance Delivery~Ground"(string=w580, regular expression="\">FSX</a>" ("정규식")) -> (before substring=w579:string)  [unwired: 1 in, 3 out]
                  n281 = Match Pattern(string=w664, regular expression="," ("정규식")) -> (before substring=w661:string, after substring=w660:string)  [unwired: 1 in, 2 out]
                  n282 = call <vilib>:"Trim Whitespace.vi"("string"=w542) -> ("trimmed string"=w544:string)  [unwired: 1 in]
                  n283 = Concatenate Strings(w575, w579) -> (w541:string)
                  n284 = Concatenate Strings(w575, w578) -> (w577:string)
                  n285 = Concatenate Strings(w575, w574) -> (w576:string)
                  n286 = local read "Destination"() -> (w584:string)
                  n287 = Match Pattern "Clearance Delivery~Ground"(string=w548, regular expression="<!" ("문자열")) -> (after substring=w697:string)  [unwired: 1 in, 3 out]
                  n288 = Concatenate Strings(w661, w660) -> (w663:string)
                  n289 = Concatenate Strings("https://flightplandatabase.com" ("url"), w544) -> (w704:string)
                  n290 = call <vilib>:"Clear Errors.vi"("error in (no error)"=w683, "specific error code to clear (0: all)"=0) -> ("error out"=w684:errorcluster)  [unwired: 4 in, 1 out]
                  n291 = call <vilib>:"Trim Whitespace.vi"("string"=w541) -> ("trimmed string"=w555:string)  [unwired: 1 in]
                  n292 = call <vilib>:"Trim Whitespace.vi"("string"=w577) -> ("trimmed string"=w540:string)  [unwired: 1 in]
                  n293 = call <vilib>:"Trim Whitespace.vi"("string"=w576) -> ("trimmed string"=w534:string)  [unwired: 1 in]
                  n294 = Decimal String To Number(string=w663) -> (number=w665:i32)  [unwired: 2 in, 1 out]
                  n295 = call <vilib>:"Trim Whitespace.vi"("string"=w704) -> ("trimmed string"=w652:string)  [unwired: 1 in]
                  n296 = call <vilib>:"Unset Busy.vi"("error in (no error)"=w684) -> ()  [unwired: 10 in, 1 out]
                  n297 = Multiply(x=w665, y=1.85) -> (x*y=w656:dbl)
                  n298 = Read from Text File(file (use dialog)=w623) -> (text=w604:string)  [unwired: 1 in, 5 out]
                  n299 = Match Pattern "Clearance Delivery~Ground"(string=w697, regular expression=" html>" ("정규식")) -> (before substring=w696:string)  [unwired: 1 in, 3 out]
                  n300 = disable-structure shown="활성화" {
                    disable-tunnel: w656 -> [w963 _]
                    frame Disabled {
                      n301 = Divide(x=w963, y=0.1041428571428571) -> (x/y=w964:dbl)
                      n302 = Multiply(x=w964, y=0.1) -> (x*y=w962:dbl)
                      n303 = Add(x=w964, y=w962) -> (x+y=w961:dbl)
                      n304 = Multiply(x=w961, y=2.204623) -> (x*y=w959:dbl)
                      n305 = To Long Integer(number=w959) -> ()  [unwired: 1 out]
                    }
                    frame Enabled {
                    }
                  }
                  n306 = call <vilib>:"GET.vi"("url"=w652) -> ("body"=w583:string, "error out"=w651:errorcluster)  [unwired: 11 in, 2 out]
                  n307 = Concatenate Strings(w633, "\\data\\RWY" ("문자열")) -> (w591:string)
                  n308 = Divide(x=w656, y=850.0) -> (x/y=w657:dbl)
                  n309 = call <vilib>:"GET.vi"("url"=w540) -> ("body"=w569:string, "error out"=w562:errorcluster)  [unwired: 11 in, 2 out]
                  n310 = call <vilib>:"GET.vi"("url"=w534) -> ("body"=w573:string, "error out"=w560:errorcluster)  [unwired: 11 in, 2 out]
                  n311 = call <vilib>:"GET.vi"("url"=w555) -> ("body"=w572:string, "error out"=w563:errorcluster)  [unwired: 11 in, 2 out]
                  n312 = Match Pattern(string=w604, regular expression=w584) -> (after substring=w605:string)  [unwired: 1 in, 3 out]
                  n313 = String To Path(string=w591) -> (path=w586:path)
                  n314 = Concatenate Strings(w584, "END;" ("정규식")) -> (w602:string)
                  n315 = Number To Decimal String(number=w657) -> (decimal integer string=w678:string)  [unwired: 1 in]
                  n316 = Equal?(x=w696, y="DOCTYPE") -> (x = y?=w655:bool)
                  n317 = Match Pattern "Clearance Delivery~Ground"(string=w583, regular expression="<!" ("문자열")) -> (after substring=w694:string)  [unwired: 1 in, 3 out]
                  n318 = Concatenate Strings(w678, "시간") -> ()  [unwired: 1 out]
                  n319 = Match Pattern(string=w605, regular expression=w602) -> (before substring=w603:string)  [unwired: 1 in, 3 out]
                  n320 = Less Or Equal?(x=w657, y=0.5) -> (x <= y?=w659:bool)
                  n321 = Match Pattern "Clearance Delivery~Ground"(string=w694, regular expression=" html>" ("정규식")) -> (before substring=w691:string)  [unwired: 1 in, 3 out]
                  n322 = call <vilib>:"Clear Errors.vi"("error in (no error)"=w563, "specific error code to clear (0: all)"=0) -> ()  [unwired: 4 in, 2 out]
                  n323 = call <vilib>:"Clear Errors.vi"("error in (no error)"=w560, "specific error code to clear (0: all)"=0) -> ()  [unwired: 4 in, 2 out]
                  n324 = call <vilib>:"Clear Errors.vi"("error in (no error)"=w562, "specific error code to clear (0: all)"=0) -> ()  [unwired: 4 in, 2 out]
                  n325 = case shown="거짓" w659 {
                    tunnel: w657 -> [w1012 w1013]
                    frame False {
                      n326 = Round To Nearest(number=w1012) -> (nearest integer value=→"time/시간":dbl)
                    }
                    frame True {
                      n327 = local write "time/시간"(w1013) -> ()
                    }
                  }
                  n328 = Equal?(x=w691, y="DOCTYPE") -> (x = y?=w570:bool)
                  n329 = Match Pattern(string=w603, regular expression="rwy" ("문자열")) -> (after substring=w600:string)  [unwired: 1 in, 3 out]
                  n330 = case shown="거짓" w655 {
                    tunnel: w548 -> [w978 _]
                    frame False {
                      w976 = "\r"
                      n331 = local read "Destination"() -> (w979:string)
                      n332 = local read "Distance"() -> (w975:string)
                      n333 = local read "departure"() -> (w981:string)
                      n334 = To Upper Case(1:w979) -> (0:w980:string)
                      n335 = To Upper Case(1:w981) -> (0:w982:string)
                      n336 = Concatenate Strings(w982, w980, ":", w976, w978, w976, "\tDistance", w976, w975, "\r", "end", "\r") -> (w983:string)
                      n337 = call <vilib>:"Application Directory.vi"() -> ("Application Directory"=w970:path)
                      n338 = Path To String(path=w970) -> (string=w968:string)
                      n339 = Build Array(w983) -> (w986:string[])
                      n340 = Concatenate Strings(w968, "\\data\\fsm-offlinedata.pbfs" ("문자열")) -> (w969:string)
                      n341 = String To Path(string=w969) -> (path=w967:path)
                      n342 = call-poly <vilib>:"Write To Spreadsheet File.vi"("delimiter (\\t)"="\\n" ("delimiter (\\t)"), "transpose? (no:F)"=FALSE, "append to file? (new file:F)"=TRUE, "1D data"=w986, "file path (dialog if empty)"=w967) -> ()  [unwired: 3 in, 1 out]
                    }
                    frame True {
                    }
                  }
                  n343 = case shown="거짓" w570 {
                    tunnel: w573 -> [w793 _]
                    frame False {
                      "PMDG" <- w793
                    }
                    frame True {
                      n344 = local write "PMDG"("찾을수 없습니다.") -> ()
                    }
                  }
                  n345 = case shown="거짓" w570 {
                    tunnel: w583 -> [w1021 _]
                    frame False {
                      "x fmc 플랜" <- w1021
                    }
                    frame True {
                      n346 = local write "x fmc 플랜"("찾을수 없습니다.") -> ()
                    }
                  }
                  n347 = case shown="참" w570 {
                    tunnel: w572 -> [w797 _]
                    frame False {
                      "FSX" <- w797
                    }
                    frame True {
                      n348 = local write "FSX"("찾을수 없습니다.") -> ()
                    }
                  }
                  n349 = Match Pattern(string=w600, regular expression="rwyand;" ("정규식")) -> (before substring=w599:string)  [unwired: 1 in, 3 out]
                  n350 = case shown="거짓" w570 {
                    tunnel: w569 -> [w795 _]
                    frame False {
                      "FS2004/FS9" <- w795
                    }
                    frame True {
                      n351 = local write "FS2004/FS9"("찾을수 없습니다.") -> ()
                    }
                  }
                  n352 = case shown="거짓" w570 {
                    tunnel: w583 -> [w1004 _]
                    frame False {
                      w998 = "\r"
                      # "xfmc-offlinedata.pbfs"
                      n353 = local read "Destination"() -> (w1000:string)
                      n354 = local read "departure"() -> (w1003:string)
                      n355 = local read "Distance"() -> (w997:string)
                      n356 = To Upper Case(1:w1000) -> (0:w1001:string)
                      n357 = To Upper Case(1:w1003) -> (0:w1002:string)
                      n358 = Concatenate Strings(w1002, w1001, ":", w1004, w998, "Distance" ("문자열"), w998, w997, "\r", "end", "\r") -> (w1005:string)
                      n359 = call <vilib>:"Application Directory.vi"() -> ("Application Directory"=w992:path)
                      n360 = Build Array(w1005) -> (w1008:string[])
                      n361 = Path To String(path=w992) -> (string=w990:string)
                      n362 = Concatenate Strings(w990, "\\data\\xfmc-offlinedata.pbfs" ("문자열")) -> (w991:string)
                      n363 = String To Path(string=w991) -> (path=w989:path)
                      n364 = call-poly <vilib>:"Write To Spreadsheet File.vi"("delimiter (\\t)"="\\n" ("delimiter (\\t)"), "transpose? (no:F)"=FALSE, "append to file? (new file:F)"=TRUE, "1D data"=w1008, "file path (dialog if empty)"=w989) -> ()  [unwired: 3 in, 1 out]
                    }
                    frame True {
                    }
                  }
                  n365 = case shown="거짓" w570 {
                    tunnel: w569 -> [w764 _]
                    frame False {
                      w758 = "\r"
                      # "fs2004_offlinedata.pbfs"
                      n366 = local read "Destination"() -> (w760:string)
                      n367 = local read "departure"() -> (w763:string)
                      n368 = local read "Distance"() -> (w757:string)
                      n369 = To Upper Case(1:w760) -> (0:w761:string)
                      n370 = To Upper Case(1:w763) -> (0:w762:string)
                      n371 = Concatenate Strings(w762, w761, ":", w764, w758, "Distance" ("문자열"), w758, w757, "\r", "end", "\r") -> (w765:string)
                      n372 = call <vilib>:"Application Directory.vi"() -> ("Application Directory"=w752:path)
                      n373 = Build Array(w765) -> (w768:string[])
                      n374 = Path To String(path=w752) -> (string=w750:string)
                      n375 = Concatenate Strings(w750, "\\data\\fs2004_offlinedata.pbfs" ("문자열")) -> (w751:string)
                      n376 = String To Path(string=w751) -> (path=w749:path)
                      n377 = call-poly <vilib>:"Write To Spreadsheet File.vi"("delimiter (\\t)"="\\n" ("delimiter (\\t)"), "transpose? (no:F)"=FALSE, "append to file? (new file:F)"=TRUE, "1D data"=w768, "file path (dialog if empty)"=w749) -> ()  [unwired: 3 in, 1 out]
                    }
                    frame True {
                    }
                  }
                  n378 = case shown="거짓" w570 {
                    tunnel: w572 -> [w786 _]
                    frame False {
                      w780 = "\r"
                      # "fsx-offlinedatapbfs"
                      n379 = local read "Destination"() -> (w782:string)
                      n380 = local read "departure"() -> (w785:string)
                      n381 = local read "Distance"() -> (w779:string)
                      n382 = To Upper Case(1:w782) -> (0:w783:string)
                      n383 = To Upper Case(1:w785) -> (0:w784:string)
                      n384 = Concatenate Strings(w784, w783, ":", w786, w780, "Distance" ("문자열"), w780, w779, "\r", "end", "\r") -> (w787:string)
                      n385 = call <vilib>:"Application Directory.vi"() -> ("Application Directory"=w774:path)
                      n386 = Build Array(w787) -> (w790:string[])
                      n387 = Path To String(path=w774) -> (string=w772:string)
                      n388 = Concatenate Strings(w772, "\\data\\fsx-offlinedata.pbfs" ("문자열")) -> (w773:string)
                      n389 = String To Path(string=w773) -> (path=w771:path)
                      n390 = call-poly <vilib>:"Write To Spreadsheet File.vi"("delimiter (\\t)"="\\n" ("delimiter (\\t)"), "transpose? (no:F)"=FALSE, "append to file? (new file:F)"=TRUE, "1D data"=w790, "file path (dialog if empty)"=w771) -> ()  [unwired: 3 in, 1 out]
                    }
                    frame True {
                    }
                  }
                  n391 = Open/Create/Replace File(file path (use dialog)=w586, operation (0:open)=T1."replace or create" ("동작(0:open)"), access (0:read/write)=enum16{"read/write", "read-only", "write-only"}."read/write" ("접근(0:읽기/쓰기)")) -> (refnum out=w594:refnum<file>, error out=w597:errorcluster)  [unwired: 3 in, 1 out]
                  n392 = call <vilib>:"Trim Whitespace.vi"("string"=w599) -> ("trimmed string"=w598:string)  [unwired: 1 in]
                  n393 = call <vilib>:"Clear Errors.vi"("error in (no error)"=w651, "specific error code to clear (0: all)"=0) -> ()  [unwired: 4 in, 2 out]
                  n394 = case shown="참" w655 {
                    tunnel: w548 -> [w1023 _]
                    frame False {
                      "fms" <- w1023
                    }
                    frame True {
                      n395 = local write "FMS 플랜"("찾을수 없습니다.") -> ()
                    }
                  }
                  n396 = Write to Text File(file (use dialog)=w594, text=w598, error in=w597) -> (refnum out=w595:refnum<file>, error out=w596:errorcluster)  [unwired: 1 in, 1 out]
                  n397 = Close File(refnum=w595, error in=w596) -> (error out=w632:errorcluster)  [unwired: 1 out]
                  n398 = Read from Text File(file (use dialog)=w586, error in=w632) -> (text=w617:string)  [unwired: 5 out]
                  n399 = case shown="거짓" w570 {
                    tunnel: w569 -> [w742 _]
                    frame False {
                      w736 = "\r"
                      # "pmdg-offlinedata..pbfs"
                      n400 = local read "Destination"() -> (w738:string)
                      n401 = local read "departure"() -> (w741:string)
                      n402 = local read "Distance"() -> (w735:string)
                      n403 = To Upper Case(1:w738) -> (0:w739:string)
                      n404 = To Upper Case(1:w741) -> (0:w740:string)
                      n405 = Concatenate Strings(w740, w739, ":", w742, w736, "Distance" ("문자열"), w736, w735, "\r", "end", "\r") -> (w743:string)
                      n406 = call <vilib>:"Application Directory.vi"() -> ("Application Directory"=w730:path)
                      n407 = Build Array(w743) -> (w746:string[])
                      n408 = Path To String(path=w730) -> (string=w728:string)
                      n409 = Concatenate Strings(w728, "\\data\\pmdg-offlinedata.pbfs" ("문자열")) -> (w729:string)
                      n410 = String To Path(string=w729) -> (path=w727:path)
                      n411 = call-poly <vilib>:"Write To Spreadsheet File.vi"("delimiter (\\t)"="\\n" ("delimiter (\\t)"), "transpose? (no:F)"=FALSE, "append to file? (new file:F)"=TRUE, "1D data"=w746, "file path (dialog if empty)"=w727) -> ()  [unwired: 3 in, 1 out]
                    }
                    frame True {
                    }
                  }
                  n412 = Spreadsheet String To Array(delimiter (Tab)="\r", format string="%d", spreadsheet string=w617) -> (array=w615:dbl[][])  [unwired: 1 out]
                  n413 = Read from Text File(file (use dialog)=w623) -> (text=w630:string)  [unwired: 1 in, 5 out]
                  n414 = local read "Destination"() -> (w624:string)
                  n415 = To Upper Case(1:w624) -> (0:w625:string)
                  n416 = Array Size(array=w615) -> (size(s)=w616:i32[])
                  n417 = Concatenate Strings(w625, "END;" ("정규식")) -> (w628:string)
                  n418 = Match Pattern(string=w630, regular expression=w625) -> (after substring=w626:string)  [unwired: 1 in, 3 out]
                  n419 = Index Array(array=w616) -> (element=w618:i32)  [unwired: 1 in]
                  n420 = call <vilib>:"Clear Errors.vi"("specific error code to clear (0: all)"=0) -> ("error out"=w612:errorcluster)  [unwired: 5 in, 1 out]
                  n421 = Match Pattern(string=w626, regular expression=w628) -> (before substring=w637:string)  [unwired: 1 in, 3 out]
                  n422 = Equal?(x=w637, y="") -> (x = y?=w634:bool)
                  n423 = Read from Text File(file (use dialog)=w586, count=w618, error in=w612) -> (text=w608:string[], error out=w610:errorcluster)  [unwired: 3 out]
                  n424 = flat-sequence {
                    tunnel: w643 -> [w910]
                    tunnel: [w909] -> w638
                    tunnel: [w908] -> w622
                    tunnel: w640 -> [w937]
                    tunnel: w639 -> [w935]
                    tunnel: w638 -> [w936]
                    tunnel: w636 -> [w934]
                    tunnel: w635 -> [w931]
                    tunnel: [w933] -> w582
                    tunnel: w634 -> [w932]
                    frame #0 {
                      (unwired) "https://flightplandatabase.com/plan/435659"
                      # "https://flightplandatabase.com/plan/425078"
                      n425 = call <vilib>:"GET.vi"("url"=w910) -> ("body"=w930:string)  [unwired: 11 in, 3 out]
                      n426 = call <vilib>:"GET.vi"("url"=w910) -> ("body"=w915:string)  [unwired: 11 in, 3 out]
                      n427 = Match Pattern(string=w930, regular expression="<h2 class=\"main-item-title\">METAR</h2>" ("정규식")) -> (after substring=w928:string)  [unwired: 1 in, 3 out]
                      n428 = Match Pattern(string=w915, regular expression="<div class=\"main-item weather-widget\" id=\"weather-to\">" ("정규식")) -> (after substring=w917:string)  [unwired: 1 in, 3 out]
                      n429 = Match Pattern(string=w928, regular expression="<br><br><a style=\"font-size: 80%\" " ("정규식")) -> (before substring=w926:string)  [unwired: 1 in, 3 out]
                      n430 = Match Pattern(string=w917, regular expression="<br><br><a style=\"font-size: 80%\" rel=\"nofollow\" href=\"" ("정규식")) -> (before substring=w919:string)  [unwired: 1 in, 3 out]
                      n431 = Match Pattern(string=w926, regular expression="<span>" ("정규식")) -> (after substring=w924:string)  [unwired: 1 in, 3 out]
                      n432 = Match Pattern(string=w919, regular expression="<span>" ("정규식")) -> (after substring=w921:string)  [unwired: 1 in, 3 out]
                      n433 = Match Pattern(string=w924, regular expression="</span>" ("정규식")) -> (before substring=w912:string)  [unwired: 1 in, 3 out]
                      n434 = Match Pattern(string=w921, regular expression="</span>" ("정규식")) -> (before substring=w908:string)  [unwired: 1 in, 3 out]
                      n435 = Concatenate Strings(w912, "\r", "-------------------------------------------------" ("문자열"), "\r", w908) -> (w909:string)
                    }
                    frame #1 {
                      n436 = case shown="참" w932 {
                        tunnel: w937 -> [w945 w955]
                        tunnel: w936 -> [w946 w954]
                        tunnel: w935 -> [w938 w953]
                        tunnel: w934 -> [_ w951]
                        tunnel: w931 -> [w941 w949]
                        tunnel: [w944 w948] -> w933
                        frame False {
                          w940 = "\r"
                          n437 = call <vilib>:"Trim Whitespace.vi"("string"=w938) -> ("trimmed string"=w939:string)  [unwired: 1 in]
                          n438 = Concatenate Strings(w941, w940, w940, w945, w940, w939) -> (w942:string)
                          n439 = call <vilib>:"Trim Whitespace.vi"("string"=w942) -> ("trimmed string"=w943:string)  [unwired: 1 in]
                          n440 = Concatenate Strings(w946, w940, "--------------frequency------------" ("문자열"), w940, w943) -> (w944:string)
                        }
                        frame True {
                          w956 = "\r"
                          n441 = call <vilib>:"Trim Whitespace.vi"("string"=w951) -> ("trimmed string"=w952:string)  [unwired: 1 in]
                          n442 = call <vilib>:"Trim Whitespace.vi"("string"=w949) -> ("trimmed string"=w950:string)  [unwired: 1 in]
                          n443 = Concatenate Strings(w952, w956, w955, w956, w950, w956, w953, w956) -> (w957:string)
                          n444 = Concatenate Strings(w954, w956, "----------------------------------------" ("문자열"), w956, w957) -> (w948:string)
                        }
                      }
                    }
                  }
                  n445 = call <vilib>:"Clear Errors.vi"("error in (no error)"=w610, "specific error code to clear (0: all)"=0) -> ()  [unwired: 4 in, 2 out]
                  n446 = Sort 1D Array(array=w608) -> (sorted array=w631:string[])
                  "활주로" <- w631
                  n447 = Array Size(array=w631) -> (size(s)=w620:i32)
                  n448 = Match Pattern(string=w622, regular expression="Z" ("정규식")) -> (after substring=w645:string)  [unwired: 1 in, 3 out]
                  n449 = Match Pattern(string=w645, regular expression="KT" ("정규식")) -> (before substring=w642:string)  [unwired: 1 in, 3 out]
                  n450 = String Subset(string=w642, length (rest)=4 ("길이(나머지)")) -> (substring=w588:string)  [unwired: 1 in]
                  n451 = for {
                    N: w620 -> [_]
                    shift-right: [w815] -> _
                    shift-left: i32[] [] -> [w819]
                    shift-right: [w802] -> _
                    shift-left: i32[] [] -> [w813]
                    tunnel: w588 -> [w800]
                    tunnel: [w803] -> w589 mode=indexing
                    tunnel: [w799] -> w587 mode=indexing
                    i -> [w820]
                    n452 = local read "활주로"() -> (w818:string[])
                    n453 = Index Array(array=w818, index=w820) -> (element=w817:string)
                    n454 = Decimal String To Number(string=w800) -> (number=w805:i32)  [unwired: 2 in, 1 out]
                    n455 = Decimal String To Number(string=w817) -> (number=w809:i32)  [unwired: 2 in, 1 out]
                    n456 = Absolute Value(x=w809) -> (abs(x)=w804:i32)
                    n457 = Subtract(x=w805, y=w804) -> (x-y=w808:i32)
                    n458 = Build Array (concatenate)(w804, w813) -> (w802:i32[])
                    n459 = Absolute Value(x=w808) -> (abs(x)=w807:i32)
                    n460 = Build Array (concatenate)(w807, w819) -> (w815:i32[])
                    n461 = Array Max & Min(array=w815) -> (min index (indices)=w814:i32)  [unwired: 3 out]
                    n462 = Sort 1D Array(array=w815) -> (sorted array=w816:i32[])
                    n463 = Reverse 1D Array(array=w816) -> ()  [unwired: 1 out]
                    n464 = Index Array(array=w802, index=w814) -> (element=w810:i32)
                    n465 = Absolute Value(x=w810) -> (abs(x)=w811:i32)
                    n466 = Index Array(array=w802, index=0 ("인덱스")) -> (element=w799:i32)
                    n467 = Divide(x=w811, y=10) -> (x/y=w806:dbl)
                    n468 = To Long Integer(number=w806) -> (32bit integer=w803:i32)
                  }
                  n469 = case shown="참" w634 {
                    tunnel: [_ w879] -> w640
                    tunnel: [w826 w878] -> w639
                    tunnel: w637 -> [w827 _]
                    tunnel: [_ "departure"] -> w636
                    tunnel: [_ " Destination"] -> w635
                    tunnel: w589 -> [w825 _]
                    tunnel: w588 -> [w823 _]
                    tunnel: w587 -> [w821 _]
                    frame False {
                      n470 = Equal?(x=w823, y="") -> (x = y?=w824:bool)
                      n471 = case shown="참" w824 {
                        tunnel: w827 -> [w841 w853]
                        tunnel: [w828 w854] -> w826
                        tunnel: w825 -> [w831 _]
                        tunnel: w821 -> [_ w851]
                        frame False {
                          w836 = "\r"
                          # "õ¬mÕüÈÓÂ œÍ%¸"
                          # "\\ÖüÈ\\¸  ÁÝÐ"
                          n472 = Index Array(array=w831, index=0 ("인덱스")) -> (element=w829:i32)
                          n473 = Number To Decimal String(number=w829) -> (decimal integer string=w842:string)  [unwired: 1 in]
                          n474 = Match Pattern(string=w841, regular expression="frequency") -> (after substring=w846:string)  [unwired: 1 in, 3 out]
                          n475 = Concatenate Strings("frequency", "and;") -> (w845:string)
                          n476 = Concatenate Strings("rwy", w842) -> (w840:string)
                          n477 = Match Pattern(string=w846, regular expression=w845) -> (before substring=w833:string)  [unwired: 1 in, 3 out]
                          n478 = Concatenate Strings(w842, "and") -> (w838:string)
                          n479 = Match Pattern(string=w841, regular expression=w840) -> (after substring=w839:string)  [unwired: 1 in, 3 out]
                          n480 = call <vilib>:"Trim Whitespace.vi"("string"=w833) -> ("trimmed string"=w832:string)  [unwired: 1 in]
                          n481 = Match Pattern(string=w839, regular expression=w838) -> (before substring=w835:string)  [unwired: 1 in, 3 out]
                          n482 = Concatenate Strings(w832, w836, "----------------RWY--------------", w836, w835) -> (w834:string)
                          n483 = call <vilib>:"Trim Whitespace.vi"("string"=w834) -> ("trimmed string"=w828:string)  [unwired: 1 in]
                        }
                        frame True {
                          w859 = "\r"
                          # "õ¬mÕüÈÓÂ œÍ%¸"
                          # "\\ÖüÈ\\¸  ÁÝÐ"
                          n484 = Index Array(array=w851, index=0 ("인덱스")) -> (element=w850:i32)
                          n485 = Number To Decimal String(number=w850) -> (decimal integer string=w864:string)  [unwired: 1 in]
                          n486 = Match Pattern(string=w853, regular expression="frequency") -> (after substring=w868:string)  [unwired: 1 in, 3 out]
                          n487 = Concatenate Strings("frequency", "and;") -> (w867:string)
                          n488 = Concatenate Strings("rwy", w864) -> (w863:string)
                          n489 = Match Pattern(string=w868, regular expression=w867) -> (before substring=w856:string)  [unwired: 1 in, 3 out]
                          n490 = Concatenate Strings(w864, "and") -> (w861:string)
                          n491 = Match Pattern(string=w853, regular expression=w863) -> (after substring=w862:string)  [unwired: 1 in, 3 out]
                          n492 = call <vilib>:"Trim Whitespace.vi"("string"=w856) -> ("trimmed string"=w855:string)  [unwired: 1 in]
                          n493 = Match Pattern(string=w862, regular expression=w861) -> (before substring=w858:string)  [unwired: 1 in, 3 out]
                          n494 = Concatenate Strings(w855, w859, "----------------RWY--------------", w859, w858) -> (w857:string)
                          n495 = call <vilib>:"Trim Whitespace.vi"("string"=w857) -> ("trimmed string"=w854:string)  [unwired: 1 in]
                        }
                      }
                    }
                    frame True {
                      (unwired) "RKPC" ("문자열")
                      (unwired) "RKSS" ("문자열")
                      n496 = local read "departure"() -> (w875:string)
                      n497 = local read "Destination"() -> (w873:string)
                      n498 = To Upper Case(1:w875) -> (0:w874:string)
                      n499 = To Upper Case(1:w873) -> (0:w872:string)
                      n500 = Concatenate Strings("http://airportnavfinder.com/airport/", w874) -> (w907:string)
                      n501 = Concatenate Strings("http://airportnavfinder.com/airport/", w872) -> (w881:string)
                      n502 = call <vilib>:"GET.vi"("url"=w907) -> ("body"=w905:string)  [unwired: 11 in, 3 out]
                      n503 = call <vilib>:"GET.vi"("url"=w881) -> ("body"=w883:string)  [unwired: 11 in, 3 out]
                      n504 = Match Pattern(string=w883, regular expression="<div class=\"boxheader\">Airport Radio Frequencies<span class=right></span></div>" ("정규식")) -> (after substring=w885:string)  [unwired: 1 in, 3 out]
                      n505 = Match Pattern(string=w905, regular expression="<div class=\"boxheader\">Airport Radio Frequencies<span class=right></span></div>" ("정규식")) -> (after substring=w903:string)  [unwired: 1 in, 3 out]
                      n506 = Match Pattern(string=w903, regular expression="</table>" ("정규식")) -> (before substring=w901:string)  [unwired: 1 in, 3 out]
                      n507 = Match Pattern(string=w885, regular expression="</table>" ("정규식")) -> (before substring=w880:string)  [unwired: 1 in, 3 out]
                      n508 = Match Pattern(string=w880, regular expression="<table border=\"0\"><tr><th nowrap align=\"right\">" ("정규식")) -> (after substring=w888:string)  [unwired: 1 in, 3 out]
                      n509 = Match Pattern(string=w901, regular expression="<table border=\"0\"><tr><th nowrap align=\"right\">" ("정규식")) -> (after substring=w899:string)  [unwired: 1 in, 3 out]
                      n510 = Match Pattern(string=w888, regular expression="</th><td>" ("정규식")) -> (before substring=w892:string, after substring=w890:string)  [unwired: 1 in, 2 out]
                      n511 = Match Pattern(string=w899, regular expression="</th><td>" ("정규식")) -> (before substring=w895:string, after substring=w897:string)  [unwired: 1 in, 2 out]
                      n512 = Match Pattern(string=w897, regular expression="</td></tr><tr><th nowrap align=\"right\">" ("정규식")) -> (before substring=w894:string)  [unwired: 1 in, 3 out]
                      n513 = Match Pattern(string=w890, regular expression="</td></tr><tr><th nowrap align=\"right\">" ("정규식")) -> (before substring=w893:string)  [unwired: 1 in, 3 out]
                      n514 = Concatenate Strings(w892, w893) -> (w878:string)
                      n515 = Concatenate Strings(w895, w894) -> (w879:string)
                    }
                  }
                  "FMS 플랜" <- w582
                }
              }
              frame 59 {
                n516 = while {
                  stop <- FALSE stop-if-true
                  w1047 = T3 1 items=["사용자 홈"=0, "사용자 데스크탑"=1, "사용자 문서"=2, "사용자 어플리케이션 데이터"=3, "사용자 환경"=4, "사용자 임시"=5, "퍼블릭 문서"=6, "퍼블릭 어플리케이션 데이터"=7, "퍼블릭 환경"=8, "퍼블릭 캐시"=13, "시스템 코어 라이브러리"=9, "시스템 설치된 라이브러리"=10, "어플리케이션 파일"=11, "부팅 볼륨 루트"=12] ("system directory type")
                  w1048 = T3 1 items=["사용자 홈"=0, "사용자 데스크탑"=1, "사용자 문서"=2, "사용자 어플리케이션 데이터"=3, "사용자 환경"=4, "사용자 임시"=5, "퍼블릭 문서"=6, "퍼블릭 어플리케이션 데이터"=7, "퍼블릭 환경"=8, "퍼블릭 캐시"=13, "시스템 코어 라이브러리"=9, "시스템 설치된 라이브러리"=10, "어플리케이션 파일"=11, "부팅 볼륨 루트"=12] ("system directory type")
                  w1049 = T3 1 items=["사용자 홈"=0, "사용자 데스크탑"=1, "사용자 문서"=2, "사용자 어플리케이션 데이터"=3, "사용자 환경"=4, "사용자 임시"=5, "퍼블릭 문서"=6, "퍼블릭 어플리케이션 데이터"=7, "퍼블릭 환경"=8, "퍼블릭 캐시"=13, "시스템 코어 라이브러리"=9, "시스템 설치된 라이브러리"=10, "어플리케이션 파일"=11, "부팅 볼륨 루트"=12] ("system directory type")
                  w1075 = "Distance" ("정규식")
                  w1111 = T3 1 items=["사용자 홈"=0, "사용자 데스크탑"=1, "사용자 문서"=2, "사용자 어플리케이션 데이터"=3, "사용자 환경"=4, "사용자 임시"=5, "퍼블릭 문서"=6, "퍼블릭 어플리케이션 데이터"=7, "퍼블릭 환경"=8, "퍼블릭 캐시"=13, "시스템 코어 라이브러리"=9, "시스템 설치된 라이브러리"=10, "어플리케이션 파일"=11, "부팅 볼륨 루트"=12] ("system directory type")
                  w1125 = T3 1 items=["사용자 홈"=0, "사용자 데스크탑"=1, "사용자 문서"=2, "사용자 어플리케이션 데이터"=3, "사용자 환경"=4, "사용자 임시"=5, "퍼블릭 문서"=6, "퍼블릭 어플리케이션 데이터"=7, "퍼블릭 환경"=8, "퍼블릭 캐시"=13, "시스템 코어 라이브러리"=9, "시스템 설치된 라이브러리"=10, "어플리케이션 파일"=11, "부팅 볼륨 루트"=12] ("system directory type")
                  # "오프라인 모드"
                  n517 = local read "Destination"() -> (w1105:string)
                  n518 = local read "departure"() -> (w1107:string)
                  n519 = call <vilib>:"Get System Directory.vi"("system directory type"=w1047) -> ("system directory"=w1064:path)  [unwired: 10 in]
                  n520 = call <vilib>:"Get System Directory.vi"("system directory type"=w1048) -> ("system directory"=w1065:path)  [unwired: 10 in]
                  n521 = call <vilib>:"Get System Directory.vi"("system directory type"=w1049) -> ("system directory"=w1074:path)  [unwired: 10 in]
                  n522 = call <vilib>:"Get System Directory.vi"("system directory type"=w1111) -> ("system directory"=w1110:path)  [unwired: 10 in]
                  n523 = call <vilib>:"Get System Directory.vi"("system directory type"=w1125) -> ("system directory"=w1126:path)  [unwired: 10 in]
                  n524 = Build Path(base path=w1064, name or relative path="pmdg-offlinedata..pbfs" ("이름 또는 상대 경로")) -> (appended path=w1062:path)
                  n525 = Build Path(base path=w1065, name or relative path="fs2004_offlinedata.pbfs" ("이름 또는 상대 경로")) -> (appended path=w1067:path)
                  n526 = Build Path(base path=w1074, name or relative path="fsx-offlinedatapbfs" ("이름 또는 상대 경로")) -> (appended path=w1072:path)
                  n527 = To Upper Case(1:w1105) -> (0:w1104:string)
                  n528 = Build Path(base path=w1110, name or relative path="fsm-offlinedata.pbfs" ("이름 또는 상대 경로")) -> (appended path=w1113:path)
                  n529 = To Upper Case(1:w1107) -> (0:w1106:string)
                  n530 = Build Path(base path=w1126, name or relative path="xfmc-offlinedata.pbfs" ("이름 또는 상대 경로")) -> (appended path=w1123:path)
                  n531 = Concatenate Strings(w1106, w1104, ":") -> (w1050:string)
                  n532 = Read from Text File(file (use dialog)=w1062) -> (refnum out=w1061:refnum<file>, text=w1051:string, error out=w1060:errorcluster)  [unwired: 3 in, 1 out]
                  n533 = Read from Text File(file (use dialog)=w1067) -> (refnum out=w1068:refnum<file>, text=w1054:string, error out=w1069:errorcluster)  [unwired: 3 in, 1 out]
                  n534 = Read from Text File(file (use dialog)=w1072) -> (refnum out=w1071:refnum<file>, text=w1057:string, error out=w1070:errorcluster)  [unwired: 3 in, 1 out]
                  n535 = Read from Text File(file (use dialog)=w1113) -> (refnum out=w1114:refnum<file>, text=w1100:string, error out=w1115:errorcluster)  [unwired: 3 in, 1 out]
                  n536 = Read from Text File(file (use dialog)=w1123) -> (refnum out=w1122:refnum<file>, text=w1076:string, error out=w1121:errorcluster)  [unwired: 3 in, 1 out]
                  n537 = Close File(refnum=w1061, error in=w1060) -> ()  [unwired: 2 out]
                  n538 = Close File(refnum=w1068, error in=w1069) -> ()  [unwired: 2 out]
                  n539 = Close File(refnum=w1071, error in=w1070) -> ()  [unwired: 2 out]
                  n540 = Close File(refnum=w1114, error in=w1115) -> ()  [unwired: 2 out]
                  n541 = Close File(refnum=w1122, error in=w1121) -> ()  [unwired: 2 out]
                  n542 = Match Pattern(string=w1076, regular expression=w1050) -> (after substring=w1103:string)  [unwired: 1 in, 3 out]
                  n543 = Match Pattern(string=w1100, regular expression=w1050) -> (after substring=w1108:string)  [unwired: 1 in, 3 out]
                  n544 = Match Pattern(string=w1108, regular expression="Distance") -> (before substring=w1109:string)  [unwired: 1 in, 3 out]
                  n545 = Match Pattern(string=w1103, regular expression=w1075) -> (before substring=w1102:string)  [unwired: 1 in, 3 out]
                  n546 = Match Pattern(string=w1051, regular expression=w1050) -> (after substring=w1052:string)  [unwired: 1 in, 3 out]
                  n547 = Match Pattern(string=w1057, regular expression=w1050) -> (after substring=w1058:string)  [unwired: 1 in, 3 out]
                  n548 = Match Pattern(string=w1054, regular expression=w1050) -> (after substring=w1056:string)  [unwired: 1 in, 3 out]
                  n549 = Match Pattern(string=w1052, regular expression="Distance") -> (before substring=w1038:string)  [unwired: 1 in, 3 out]
                  n550 = Match Pattern(string=w1058, regular expression="Distance") -> (before substring=w1044:string)  [unwired: 1 in, 3 out]
                  n551 = Match Pattern(string=w1056, regular expression="Distance") -> (before substring=w1041:string)  [unwired: 1 in, 3 out]
                  n552 = Match Pattern(string=w1076, regular expression=w1075) -> (after substring=w1099:string)  [unwired: 1 in, 3 out]
                  n553 = Match Pattern(string=w1099, regular expression="end" ("정규식")) -> (before substring=w1089:string)  [unwired: 1 in, 3 out]
                  n554 = Equal?(x=w1102, y="") -> (x = y?=w1120:bool)
                  n555 = call <vilib>:"Trim Whitespace.vi"("string"=w1089) -> ("trimmed string"=w1095:string)  [unwired: 1 in]
                  n556 = Match Pattern "time/fuel"(string=w1095, regular expression="nm" ("정규식")) -> (before substring=w1091:string)  [unwired: 1 in, 3 out]
                  n557 = Match Pattern(string=w1091, regular expression="," ("정규식")) -> (before substring=w1093:string, after substring=w1094:string)  [unwired: 1 in, 2 out]
                  n558 = Concatenate Strings(w1093, w1094) -> (w1092:string)
                  n559 = Decimal String To Number(string=w1092) -> (number=w1080:i32)  [unwired: 2 in, 1 out]
                  n560 = Multiply(x=w1080, y=1.85) -> (x*y=w1079:dbl)
                  n561 = Divide(x=w1079, y=850.0) -> (x/y=w1077:dbl)
                  n562 = Equal?(x=w1038, y="") -> (x = y?=w1040:bool)
                  n563 = Equal?(x=w1044, y="") -> (x = y?=w1046:bool)
                  n564 = Equal?(x=w1041, y="") -> (x = y?=w1042:bool)
                  n565 = Equal?(x=w1109, y="") -> (x = y?=w1117:bool)
                  n566 = case shown="거짓" w1040 {
                    tunnel: w1038 -> [w1128 _]
                    frame False {
                      n567 = local write "PMDG"(w1128) -> ()
                    }
                    frame True {
                      n568 = local write "x fmc 플랜"("오프라인  데이터에 없습니다. !" ("메시지")) -> ()
                    }
                  }
                  n569 = case shown="거짓" w1046 {
                    tunnel: w1044 -> [w1132 _]
                    frame False {
                      n570 = local write "FSX"(w1132) -> ()
                    }
                    frame True {
                      n571 = local write "x fmc 플랜"("오프라인  데이터에 없습니다. !" ("메시지")) -> ()
                    }
                  }
                  n572 = case shown="거짓" w1042 {
                    tunnel: w1041 -> [w1130 _]
                    frame False {
                      n573 = local write "FS2004/FS9"(w1130) -> ()
                    }
                    frame True {
                      n574 = local write "x fmc 플랜"("오프라인  데이터에 없습니다. !" ("메시지")) -> ()
                    }
                  }
                  n575 = case shown="거짓" w1117 {
                    tunnel: w1109 -> [w1134 _]
                    frame False {
                      n576 = local write "FMS 플랜"(w1134) -> ()
                    }
                    frame True {
                      n577 = local write "x fmc 플랜"("오프라인  데이터에 없습니다. !" ("메시지")) -> ()
                    }
                  }
                  n578 = Divide(x=w1079, y=0.1041428571428571) -> (x/y=w1083:dbl)
                  n579 = Multiply(x=w1083, y=0.1) -> (x*y=w1084:dbl)
                  n580 = Add(x=w1083, y=w1084) -> (x+y=w1085:dbl)
                  n581 = Multiply(x=w1085, y=2.204623) -> (x*y=w1087:dbl)
                  n582 = To Long Integer(number=w1087) -> (32bit integer=w1078:i32)
                  n583 = case shown="거짓" w1120 {
                    tunnel: w1102 -> [w1140 _]
                    tunnel: w1078 -> [_ _]
                    tunnel: w1077 -> [w1136 _]
                    tunnel: w1077 -> [w1137 _]
                    frame False {
                      n584 = Less Or Equal?(x=w1137, y=0.5) -> (x <= y?=w1139:bool)
                      n585 = local write "x fmc 플랜"(w1140) -> ()
                      n586 = case shown="거짓" w1139 {
                        tunnel: w1136 -> [w1141 w1143]
                        frame False {
                          n587 = Round To Nearest(number=w1141) -> (nearest integer value=w1142:dbl)
                          n588 = local write "time/시간"(w1142) -> ()
                        }
                        frame True {
                          n589 = local write "time/시간"(w1143) -> ()
                        }
                      }
                    }
                    frame True {
                      n590 = local write "x fmc 플랜"("오프라인  데이터에 없습니다. !" ("메시지")) -> ()
                    }
                  }
                }
              }
            }
          }
        }
        n591 = Wait Until Next ms Multiple(millisecond multiple=u32 100 ("ms 배수")) -> ()  [unwired: 1 out]
        n592 = local read "FS2004/FS9"() -> (w215:string)
        n593 = local read "FS2004/FS9"() -> (w209:string)
        n594 = local read "x fmc 플랜"() -> (w192:string)
        n595 = local read "x fmc 플랜"() -> (w254:string)
        n596 = local read "x fmc 플랜"() -> (w260:string)
        n597 = local read "FMS 플랜"() -> (w249:string)
        n598 = local read "FMS 플랜"() -> (w258:string)
        n599 = local read "FSX"() -> (w194:string)
        n600 = local read "FSX"() -> (w218:string)
        n601 = local read "FSX"() -> (w211:string)
        n602 = local read "x fmc 플랜"() -> (w236:string)
        n603 = local read "FMS 플랜"() -> (w232:string)
        n604 = local read "FS2004/FS9"() -> (w203:string)
        n605 = local read "FS2004/FS9"() -> (w196:string)
        n606 = local read "FSX"() -> (w206:string)
        n607 = Equal?(x=w215, y="") -> (x = y?=w213:bool)
        n608 = Equal?(x=w209, y="찾을수 없습니다.") -> (x = y?=w208:bool)
        n609 = Equal?(x=w196, y="오프라인  데이터에 없습니다. !") -> (x = y?=w190:bool)
        n610 = Equal?(x=w194, y="") -> (x = y?=w191:bool)
        n611 = Equal?(x=w218, y="") -> (x = y?=w214:bool)
        n612 = Equal?(x=w211, y="찾을수 없습니다.") -> (x = y?=w207:bool)
        n613 = Equal?(x=w192, y="찾을수 없습니다.") -> (x = y?=w188:bool)
        n614 = Equal?(x=w203, y="오프라인  데이터에 없습니다. !") -> (x = y?=w205:bool)
        n615 = Equal?(x=w254, y="") -> (x = y?=w256:bool)
        n616 = Equal?(x=w260, y="찾을수 없습니다.") -> (x = y?=w261:bool)
        n617 = Equal?(x=w206, y="오프라인  데이터에 없습니다. !") -> (x = y?=w204:bool)
        n618 = Equal?(x=w249, y="") -> (x = y?=w255:bool)
        n619 = Equal?(x=w258, y="찾을수 없습니다.") -> (x = y?=w262:bool)
        n620 = Equal?(x=w236, y="오프라인  데이터에 없습니다. !") -> (x = y?=w234:bool)
        n621 = Equal?(x=w232, y="오프라인  데이터에 없습니다. !") -> (x = y?=w235:bool)
        n622 = Or(x=w214, y=w213) -> (x .or. y?=w199:bool)
        n623 = And(x=w207, y=w208) -> (x .and. y?=w200:bool)
        n624 = Or(x=w204, y=w205) -> (x .or. y?=w198:bool)
        n625 = Or(x=w255, y=w256) -> (x .or. y?=w248:bool)
        n626 = And(x=w262, y=w261) -> (x .and. y?=w251:bool)
        n627 = And(x=w191, y=w190) -> (x .and. y?=w189:bool)
        n628 = Or(x=w235, y=w234) -> (x .or. y?=w233:bool)
        n629 = And(x=w189, y=w188) -> (x .and. y?=w187:bool)
        n630 = Compound Arithmetic op=OR(w251, w248, w233, w200, w199, w198, w187) -> (w250:bool)
        n631 = case shown="거짓" w250 {
          frame False {
            n632 = local read "x fmc 플랜"() -> (w1168:string)
            n633 = case shown="참" "?" {
              tunnel: w1168 -> [_ w1257]
              frame False {
              }
              frame True {
                (unwired) TRUE ("create directory if not found? (F)")
                n634 = local read "Destination"() -> (w1264:string)
                n635 = local read "departure"() -> (w1265:string)
                n636 = To Upper Case(1:w1265) -> (0:w1256:string)
                n637 = To Upper Case(1:w1264) -> (0:w1263:string)
                n638 = Concatenate Strings(w1256, w1263, ".FPL" ("문자열")) -> (w1268:string)
                n639 = Build Path(base path="저장 경로", name or relative path=w1268) -> (appended path=w1271:path)
                n640 = Open/Create/Replace File(file path (use dialog)=w1271, operation (0:open)=T1."open or create" ("동작(0:open)"), access (0:read/write)=enum16{"read/write", "read-only", "write-only"}."read/write" ("접근(0:읽기/쓰기)")) -> (refnum out=w1273:refnum<file>, error out=w1272:errorcluster)  [unwired: 3 in, 1 out]
                n641 = Write to Text File(file (use dialog)=w1273, text=w1257, error in=w1272) -> (refnum out=w1260:refnum<file>, error out=w1262:errorcluster)  [unwired: 1 in, 1 out]
                n642 = call <vilib>:"Clear Errors.vi"("error in (no error)"=w1262, "specific error code to clear (0: all)"=0) -> ("error out"=w1261:errorcluster)  [unwired: 4 in, 1 out]
                n643 = Close File(refnum=w1260, error in=w1261) -> (error out=w1258:errorcluster)  [unwired: 1 out]
                n644 = call <vilib>:"Clear Errors.vi"("error in (no error)"=w1258) -> ()  [unwired: 5 in, 2 out]
              }
            }
            n645 = local read "FS2004/FS9"() -> (w1165:string)
            n646 = case shown="거짓" "?" {
              tunnel: [_ w1172] -> _
              tunnel: w1165 -> [_ w1172]
              frame False {
              }
              frame True {
                n647 = local read "Destination"() -> (w1185:string)
                n648 = local read "departure"() -> (w1184:string)
                n649 = To Upper Case(1:w1185) -> (0:w1176:string)
                n650 = To Upper Case(1:w1184) -> (0:w1178:string)
                n651 = local read "저장 경로"() -> (w1180:path)
                n652 = Concatenate Strings(w1178, "-" ("문자열"), w1176, "_" ("문자열"), "GPS" ("문자열"), ".PLN" ("문자열")) -> (w1186:string)
                n653 = Build Path(base path=w1180, name or relative path=w1186) -> (appended path=w1189:path)
                n654 = Open/Create/Replace File(file path (use dialog)=w1189, operation (0:open)=T1."open or create" ("동작(0:open)"), access (0:read/write)=enum16{"read/write", "read-only", "write-only"}."read/write" ("접근(0:읽기/쓰기)")) -> (refnum out=w1192:refnum<file>, error out=w1191:errorcluster)  [unwired: 3 in, 1 out]
                n655 = Write to Text File(file (use dialog)=w1192, text=w1172, error in=w1191) -> (refnum out=w1190:refnum<file>, error out=w1183:errorcluster)  [unwired: 1 in, 1 out]
                n656 = call <vilib>:"Clear Errors.vi"("error in (no error)"=w1183, "specific error code to clear (0: all)"=0) -> ("error out"=w1182:errorcluster)  [unwired: 4 in, 1 out]
                n657 = Close File(refnum=w1190, error in=w1182) -> (error out=w1179:errorcluster)  [unwired: 1 out]
                n658 = call <vilib>:"Clear Errors.vi"("error in (no error)"=w1179) -> ()  [unwired: 5 in, 2 out]
              }
            }
            n659 = local read "PMDG"() -> (w1166:string)
            n660 = case shown="거짓" "?" {
              tunnel: [_ w1193] -> _
              tunnel: w1166 -> [_ w1193]
              frame False {
              }
              frame True {
                n661 = local read "Destination"() -> (w1206:string)
                n662 = local read "departure"() -> (w1205:string)
                n663 = To Upper Case(1:w1206) -> (0:w1197:string)
                n664 = To Upper Case(1:w1205) -> (0:w1199:string)
                n665 = local read "저장 경로"() -> (w1201:path)
                n666 = Concatenate Strings(w1199, "-" ("문자열"), w1197, "_" ("문자열"), "GPS" ("문자열"), ".RTE" ("문자열")) -> (w1207:string)
                n667 = Build Path(base path=w1201, name or relative path=w1207) -> (appended path=w1210:path)
                n668 = Open/Create/Replace File(file path (use dialog)=w1210, operation (0:open)=T1."open or create" ("동작(0:open)"), access (0:read/write)=enum16{"read/write", "read-only", "write-only"}."read/write" ("접근(0:읽기/쓰기)")) -> (refnum out=w1213:refnum<file>, error out=w1212:errorcluster)  [unwired: 3 in, 1 out]
                n669 = Write to Text File(file (use dialog)=w1213, text=w1193, error in=w1212) -> (refnum out=w1211:refnum<file>, error out=w1204:errorcluster)  [unwired: 1 in, 1 out]
                n670 = call <vilib>:"Clear Errors.vi"("error in (no error)"=w1204, "specific error code to clear (0: all)"=0) -> ("error out"=w1203:errorcluster)  [unwired: 4 in, 1 out]
                n671 = Close File(refnum=w1211, error in=w1203) -> (error out=w1200:errorcluster)  [unwired: 1 out]
                n672 = call <vilib>:"Clear Errors.vi"("error in (no error)"=w1200) -> ()  [unwired: 5 in, 2 out]
              }
            }
            n673 = local read "FSX"() -> (w1167:string)
            n674 = case shown="거짓" "?" {
              tunnel: [_ w1214] -> _
              tunnel: w1167 -> [_ w1214]
              frame False {
              }
              frame True {
                n675 = local read "Destination"() -> (w1227:string)
                n676 = local read "departure"() -> (w1226:string)
                n677 = To Upper Case(1:w1227) -> (0:w1218:string)
                n678 = To Upper Case(1:w1226) -> (0:w1220:string)
                n679 = local read "저장 경로"() -> (w1222:path)
                n680 = Concatenate Strings(w1220, "-" ("문자열"), w1218, "_" ("문자열"), "GPS" ("문자열"), ".PLN" ("문자열")) -> (w1228:string)
                n681 = Build Path(base path=w1222, name or relative path=w1228) -> (appended path=w1231:path)
                n682 = Open/Create/Replace File(file path (use dialog)=w1231, operation (0:open)=T1."open or create" ("동작(0:open)"), access (0:read/write)=enum16{"read/write", "read-only", "write-only"}."read/write" ("접근(0:읽기/쓰기)")) -> (refnum out=w1234:refnum<file>, error out=w1233:errorcluster)  [unwired: 3 in, 1 out]
                n683 = Write to Text File(file (use dialog)=w1234, text=w1214, error in=w1233) -> (refnum out=w1232:refnum<file>, error out=w1225:errorcluster)  [unwired: 1 in, 1 out]
                n684 = call <vilib>:"Clear Errors.vi"("error in (no error)"=w1225, "specific error code to clear (0: all)"=0) -> ("error out"=w1224:errorcluster)  [unwired: 4 in, 1 out]
                n685 = Close File(refnum=w1232, error in=w1224) -> (error out=w1221:errorcluster)  [unwired: 1 out]
                n686 = call <vilib>:"Clear Errors.vi"("error in (no error)"=w1221) -> ()  [unwired: 5 in, 2 out]
              }
            }
            n687 = local read "fms"() -> (w1170:string)
            n688 = case shown="거짓" "?" {
              tunnel: w1170 -> [_ w1250]
              frame False {
              }
              frame True {
                n689 = local read "Destination"() -> (w1247:string)
                n690 = local read "departure"() -> (w1246:string)
                n691 = To Upper Case(1:w1247) -> (0:w1238:string)
                n692 = To Upper Case(1:w1246) -> (0:w1240:string)
                n693 = local read "저장 경로"() -> (w1242:path)
                n694 = Concatenate Strings(w1240, "-" ("문자열"), w1238, "_" ("문자열"), "GPS" ("문자열"), ".FMS" ("문자열")) -> (w1248:string)
                n695 = Build Path(base path=w1242, name or relative path=w1248) -> (appended path=w1252:path)
                n696 = Open/Create/Replace File(file path (use dialog)=w1252, operation (0:open)=T1."open or create" ("동작(0:open)"), access (0:read/write)=enum16{"read/write", "read-only", "write-only"}."read/write" ("접근(0:읽기/쓰기)")) -> (refnum out=w1255:refnum<file>, error out=w1254:errorcluster)  [unwired: 3 in, 1 out]
                n697 = Write to Text File(file (use dialog)=w1255, text=w1250, error in=w1254) -> (refnum out=w1253:refnum<file>, error out=w1245:errorcluster)  [unwired: 1 in, 1 out]
                n698 = call <vilib>:"Clear Errors.vi"("error in (no error)"=w1245, "specific error code to clear (0: all)"=0) -> ("error out"=w1244:errorcluster)  [unwired: 4 in, 1 out]
                n699 = Close File(refnum=w1253, error in=w1244) -> (error out=w1241:errorcluster)  [unwired: 1 out]
                n700 = call <vilib>:"Clear Errors.vi"("error in (no error)"=w1241) -> ()  [unwired: 5 in, 2 out]
              }
            }
          }
          frame True {
          }
        }
        n701 = event shown="[0] 타임아웃" {
          selector: _ -> [_ _]
          dyn-events: _ -> [_ _]
          timeout: 10 -> [_ _]
          tunnel: [_ w264] -> w221
          event Timeout {
            n702 = event-data() -> ()  [unwired: 1 in, 3 out]
          }
          event Panel Close? {
            w264 = FALSE ("버림?")
            n703 = event-data() -> ()  [unwired: 1 in, 3 out]
            n704 = Quit LabVIEW(quit? (T)=TRUE ("종료? (참)")) -> ()
            n705 = event-data("Discard?"=w264) -> ()  [unwired: 1 in, 1 out]
          }
        }
        n706 = disable-structure shown="활성화" {
          frame Disabled {
            w1148 = T3 3 items=["사용자 홈"=0, "사용자 데스크탑"=1, "사용자 문서"=2, "사용자 어플리케이션 데이터"=3, "사용자 환경"=4, "사용자 임시"=5, "퍼블릭 문서"=6, "퍼블릭 어플리케이션 데이터"=7, "퍼블릭 환경"=8, "퍼블릭 캐시"=13, "시스템 코어 라이브러리"=9, "시스템 설치된 라이브러리"=10, "어플리케이션 파일"=11, "부팅 볼륨 루트"=12] ("system directory type")
            n707 = call <vilib>:"Get System Directory.vi"("create directory if not found? (F)"=TRUE, "system directory type"=w1148) -> ("system directory"=w1149:path)  [unwired: 9 in]
            n708 = Build Path(base path=w1149, name or relative path="number.pbfs" ("이름 또는 상대 경로")) -> (appended path=w1154:path)
            n709 = Open/Create/Replace File(file path (use dialog)=w1154, operation (0:open)=T1."open or create" ("동작(0:open)"), access (0:read/write)=enum16{"read/write", "read-only", "write-only"}."write-only" ("접근(0:읽기/쓰기)")) -> (refnum out=w1157:refnum<file>, error out=w1146:errorcluster)  [unwired: 3 in, 1 out]
            n710 = call <vilib>:"Clear Errors.vi"("error in (no error)"=w1146) -> ("error out"=w1145:errorcluster)  [unwired: 5 in, 1 out]
            n711 = Write to Text File(file (use dialog)=w1157, text="1" ("텍스트"), error in=w1145) -> (refnum out=w1158:refnum<file>, error out=w1159:errorcluster)  [unwired: 1 in, 1 out]
            n712 = call <vilib>:"Clear Errors.vi"("error in (no error)"=w1159, "specific error code to clear (0: all)"=0) -> ("error out"=w1160:errorcluster)  [unwired: 4 in, 1 out]
            n713 = Close File(refnum=w1158, error in=w1160) -> (error out=w1151:errorcluster)  [unwired: 1 out]
            n714 = call <vilib>:"Clear Errors.vi"("error in (no error)"=w1151, "specific error code to clear (0: all)"=0) -> ()  [unwired: 4 in, 2 out]
          }
          frame Enabled {
          }
        }
        n715 = for {
          N: 1 -> [_]
          n716 = call <vilib>:"Application Directory.vi"() -> ("Application Directory"=w267:path)
          n717 = Path To String(path=w267) -> (string=w269:string)
          n718 = Concatenate Strings(w269, "\\data\\location.pbfs" ("문자열")) -> (w268:string)
          n719 = String To Path(string=w268) -> (path=w265:path)
          n720 = call <vilib>:"Open Config Data.vi"("create file if necessary (T)"=TRUE, "configuration file path"=w265) -> ("error out"=w272:errorcluster, "refnum"=w273:T2)  [unwired: 7 in, 1 out]
          n721 = call-poly <vilib>:"Write Key.vi"("section"="count", "error in (no error)"=w272, "value"="1", "key"="location", "refnum"=w273) -> ("error out"=w275:errorcluster, "refnum out"=w274:T2)  [unwired: 4 in, 1 out]
          n722 = call <vilib>:"Close Config Data.vi"("error in (no error)"=w275, "write file if changed (T)"=TRUE, "refnum"=w274) -> ()  [unwired: 7 in, 2 out]
        }
        n723 = call <vilib>:"Application Directory.vi"() -> ("Application Directory"=w226:path)
        n724 = Path To String(path=w226) -> (string=w224:string)
        n725 = local read "저장 경로"() -> (w240:path)
        n726 = Concatenate Strings(w224, "\\data\\location.pbfs" ("문자열")) -> (w225:string)
        n727 = String To Path(string=w225) -> (path=w223:path)
        n728 = call <vilib>:"Open Config Data.vi"("create file if necessary (T)"=TRUE, "configuration file path"=w223) -> ("error out"=w246:errorcluster, "refnum"=w245:T2)  [unwired: 7 in, 1 out]
        n729 = call-poly <vilib>:"Write Key.vi"("section"="location", "error in (no error)"=w246, "value"=w240, "key"="location", "refnum"=w245) -> ("error out"=w243:errorcluster, "refnum out"=w244:T2)  [unwired: 4 in, 1 out]
        n730 = call <vilib>:"Close Config Data.vi"("error in (no error)"=w243, "write file if changed (T)"=TRUE, "refnum"=w244) -> ()  [unwired: 7 in, 2 out]
        n731 = control-ref of="This VI"() -> (w220:refnum<vi>)
      }
      n732 = while {
        tunnel: w140 -> [w143]
        stop <- FALSE stop-if-true
        n733 = event shown="[3] \"피드백\": 마우스 다운" {
          selector: _ -> [_ _ _ _]
          dyn-events: _ -> [_ _ _ _]
          timeout: 10 -> [_ _ _ _]
          tunnel: w143 -> [_ w146 _ _]
          event Timeout {
            n734 = event-data() -> ()  [unwired: 1 in, 3 out]
          }
          event "ATC": Mouse Down {
            n735 = event-data() -> ()  [unwired: 1 in, 8 out]
            n736 = case shown="거짓" w146 {
              frame False {
                w156 = 128  # call and forget
                n737 = vi-ref "ATCcont.vi"() -> (w149:refnum<vi>)
                n738 = property class="VI"(reference=w149) -> (error out=w150:errorcluster, "Path"=w151:path)  [unwired: 1 in, 1 out]
                n739 = Open VI Reference(type specifier VI Refnum (for type only)=refnum<vi> refnum, vi path=w151, options=w156, error in (no error)=w150) -> (vi reference=w148:refnum<vi>, error out=w154:errorcluster)  [unwired: 2 in]
                n740 = call-by-ref "Start Asynchronous Call"(reference=w148, error in=w154) -> (reference out=w147:refnum<vi>, error out=w153:errorcluster)  [unwired: 12 in]
                n741 = Close Reference(reference=w147, error in (no error)=w153) -> (error out=w152:errorcluster)
                n742 = call <vilib>:"Simple Error Handler.vi"("error in (no error)"=w152) -> ()  [unwired: 4 in, 5 out]
              }
              frame True {
                w166 = 128  # call and forget
                n743 = vi-ref "ATCpilot.vi"() -> (w159:refnum<vi>)
                n744 = property class="VI"(reference=w159) -> (error out=w160:errorcluster, "Path"=w161:path)  [unwired: 1 in, 1 out]
                n745 = Open VI Reference(type specifier VI Refnum (for type only)=refnum<vi> refnum, vi path=w161, options=w166, error in (no error)=w160) -> (vi reference=w158:refnum<vi>, error out=w164:errorcluster)  [unwired: 2 in]
                n746 = call-by-ref "Start Asynchronous Call"(reference=w158, error in=w164) -> (reference out=w157:refnum<vi>, error out=w163:errorcluster)  [unwired: 12 in]
                n747 = Close Reference(reference=w157, error in (no error)=w163) -> (error out=w162:errorcluster)
                n748 = call <vilib>:"Simple Error Handler.vi"("error in (no error)"=w162) -> ()  [unwired: 4 in, 5 out]
              }
            }
          }
          event "도움말": Mouse Down {
            w176 = 128  # call and forget
            n749 = event-data() -> ()  [unwired: 1 in, 8 out]
            n750 = vi-ref "rpopup.vi"() -> (w169:refnum<vi>)
            n751 = property class="VI"(reference=w169) -> (error out=w170:errorcluster, "Path"=w171:path)  [unwired: 1 in, 1 out]
            n752 = Open VI Reference(type specifier VI Refnum (for type only)=refnum<vi> refnum, vi path=w171, options=w176, error in (no error)=w170) -> (vi reference=w168:refnum<vi>, error out=w174:errorcluster)  [unwired: 2 in]
            n753 = call-by-ref "Start Asynchronous Call"(reference=w168, error in=w174) -> (reference out=w167:refnum<vi>, error out=w173:errorcluster)  [unwired: 12 in]
            n754 = Close Reference(reference=w167, error in (no error)=w173) -> (error out=w172:errorcluster)
            n755 = call <vilib>:"Simple Error Handler.vi"("error in (no error)"=w172) -> ()  [unwired: 4 in, 5 out]
          }
          event "피드백": Mouse Down {
            w186 = 128  # call and forget
            n756 = event-data() -> ()  [unwired: 1 in, 8 out]
            n757 = vi-ref "Feed.vi"() -> (w179:refnum<vi>)
            n758 = property class="VI"(reference=w179) -> (error out=w180:errorcluster, "Path"=w181:path)  [unwired: 1 in, 1 out]
            n759 = Open VI Reference(type specifier VI Refnum (for type only)=refnum<vi> refnum, vi path=w181, options=w186, error in (no error)=w180) -> (vi reference=w178:refnum<vi>, error out=w184:errorcluster)  [unwired: 2 in]
            n760 = call-by-ref "Start Asynchronous Call"(reference=w178, error in=w184) -> (reference out=w177:refnum<vi>, error out=w183:errorcluster)  [unwired: 12 in]
            n761 = Close Reference(reference=w177, error in (no error)=w183) -> (error out=w182:errorcluster)
            n762 = call <vilib>:"Simple Error Handler.vi"("error in (no error)"=w182) -> ()  [unwired: 4 in, 5 out]
          }
        }
      }
      n763 = invoke class="VI" method="FP.Close"(reference=w139) -> (reference out=w138:refnum<vi>)  [unwired: 2 in, 2 out]
    }
  }
  n764 = flat-sequence {
    frame #0 {
      w1275 = i32[] array[125464 elements] ("시")
      n765 = local write "시간"("" ("시간")) -> ()
      n766 = local write "분"(w1275) -> ()
      n767 = local write "초"(w1275) -> ()
      n768 = local write "시"(w1275) -> ()
    }
    frame #1 {
      n769 = while {
        shift-right: [w1305] -> _
        shift-left: i32[] [] -> [w1307]
        shift-right: [w1303] -> _
        shift-left: i32[] [] -> [w1338]
        shift-right: [w1301] -> _
        shift-left: i32[] [] -> [w1339]
        shift-right: [w1292] -> _
        shift-left: string[] [] -> [w1290]
        stop <- FALSE stop-if-true
        # "현재시간 출력"
        n770 = call "new현재시간(SubVI).vi"() -> ("분 문자열"=w1285:string, "시 문자열"=w1284:string, "초 문자열"=w1281:string)  [unwired: 3 in, 6 out]
        n771 = Wait Until Next ms Multiple(millisecond multiple=u32 200 ("ms 배수")) -> ()  [unwired: 1 out]
        n772 = case shown="거짓" "확인 버튼 2" {
          tunnel: [_ w1378] -> w1337
          tunnel: [_ w1377] -> w1332
          tunnel: [_ w1376] -> w1334
          frame False {
          }
          frame True {
            n773 = call "new현재시간(SubVI).vi"() -> ("분"=w1376:i32, "시"=w1377:i32, "분 문자열"=w1380:string, "시 문자열"=w1381:string, "초"=w1378:i32, "초 문자열"=w1379:string)  [unwired: 3 in, 3 out]
            n774 = Concatenate Strings(w1381, "hour" ("문자열"), w1380, "minute" ("문자열"), w1379, "second" ("문자열")) -> ()  [unwired: 1 out]
          }
        }
        n775 = Concatenate Strings(w1284, "hour" ("문자열"), w1285, "minute" ("문자열"), w1281, "second" ("문자열")) -> (→"시간 2":string)
        n776 = event shown="[0] 타임아웃" {
          selector: _ -> [_ _]
          dyn-events: _ -> [_ _]
          timeout: 0 -> [_ _]
          event Timeout {
            n777 = event-data() -> ()  [unwired: 1 in, 3 out]
          }
          event "기록": Mouse Down {
            w1350 = 128  # call and forget
            n778 = event-data() -> ()  [unwired: 1 in, 4 out]
            n779 = vi-ref "Flight time.vi"() -> (w1343:refnum<vi>)
            n780 = property class="VI"(reference=w1343) -> (error out=w1344:errorcluster, "Path"=w1345:path)  [unwired: 1 in, 1 out]
            n781 = Open VI Reference(type specifier VI Refnum (for type only)=refnum<vi> refnum, vi path=w1345, options=w1350, error in (no error)=w1344) -> (vi reference=w1342:refnum<vi>, error out=w1348:errorcluster)  [unwired: 2 in]
            n782 = call-by-ref "Start Asynchronous Call"(reference=w1342, error in=w1348) -> (reference out=w1341:refnum<vi>, error out=w1347:errorcluster)  [unwired: 12 in]
            n783 = Close Reference(reference=w1341, error in (no error)=w1347) -> (error out=w1346:errorcluster)
            n784 = call <vilib>:"Simple Error Handler.vi"("error in (no error)"=w1346) -> ()  [unwired: 4 in, 5 out]
          }
        }
        n785 = local read "시"() -> (w1310:i32[])
        n786 = local read "분"() -> (w1309:i32[])
        n787 = local read "초"() -> (w1308:i32[])
        n788 = Index Array(array=w1310, index=0 ("인덱스")) -> (element=w1322:i32)
        n789 = Index Array(array=w1310, index=1 ("인덱스")) -> (element=w1319:i32)
        n790 = Index Array(array=w1309, index=0 ("인덱스")) -> (element=w1316:i32)
        n791 = Index Array(array=w1309, index=1 ("인덱스")) -> (element=w1315:i32)
        n792 = Index Array(array=w1308, index=0 ("인덱스")) -> (element=w1312:i32)
        n793 = Index Array(array=w1308, index=1 ("인덱스")) -> (element=w1311:i32)
        n794 = Subtract(x=w1312, y=w1311) -> (x-y=w1294:i32)
        n795 = Subtract(x=w1316, y=w1315) -> (x-y=w1296:i32)
        n796 = Subtract(x=w1322, y=w1319) -> (x-y=w1298:i32)
        n797 = Equal?(x=w1337, y=0) -> (x = y?=w1331:bool)
        n798 = Equal?(x=w1332, y=0) -> (x = y?=w1329:bool)
        n799 = Equal?(x=w1334, y=0) -> (x = y?=w1330:bool)
        n800 = Absolute Value(x=w1294) -> (abs(x)=w1293:i32)
        n801 = Absolute Value(x=w1298) -> (abs(x)=w1297:i32)
        n802 = Absolute Value(x=w1296) -> (abs(x)=w1295:i32)
        n803 = case shown="참" w1331 {
          tunnel: w1339 -> [w1374 w1375]
          tunnel: w1337 -> [w1373 _]
          tunnel: [w1372 w1375] -> w1302
          frame False {
            n804 = Build Array (concatenate)(w1373, w1374) -> (w1372:i32[])
            "초" <- w1372
          }
          frame True {
          }
        }
        n805 = case shown="참" w1329 {
          tunnel: w1307 -> [w1366 w1367]
          tunnel: w1332 -> [w1365 _]
          tunnel: [w1364 w1367] -> w1306
          frame False {
            n806 = Build Array (concatenate)(w1365, w1366) -> (w1364:i32[])
            "시" <- w1364
          }
          frame True {
          }
        }
        n807 = case shown="참" w1330 {
          tunnel: w1338 -> [w1370 w1371]
          tunnel: w1334 -> [w1369 _]
          tunnel: [w1368 w1371] -> w1304
          frame False {
            n808 = Build Array (concatenate)(w1369, w1370) -> (w1368:i32[])
            "분" <- w1368
          }
          frame True {
          }
        }
        n809 = Number To Decimal String(number=w1297) -> (decimal integer string=w1328:string)  [unwired: 1 in]
        n810 = Number To Decimal String(number=w1295) -> (decimal integer string=w1326:string)  [unwired: 1 in]
        n811 = Number To Decimal String(number=w1293) -> (decimal integer string=w1324:string)  [unwired: 1 in]
        n812 = Concatenate Strings(w1328, "hour" ("문자열"), w1326, "minute" ("문자열"), w1324, "second" ("문자열")) -> (w1291:string)
        n813 = case shown="거짓" "초기화 2" {
          tunnel: w1306 -> [w1361 _]
          tunnel: [w1361 w1362] -> w1305
          tunnel: w1304 -> [w1360 _]
          tunnel: [w1360 w1362] -> w1303
          tunnel: w1302 -> [w1359 _]
          tunnel: [w1359 w1362] -> w1301
          tunnel: w1291 -> [w1358 _]
          tunnel: [w1358 ""] -> w1300
          frame False {
          }
          frame True {
            w1362 = i32[] array[125464 elements] ("시")
            n814 = local write "분"(w1362) -> ()
            n815 = local write "초"(w1362) -> ()
            n816 = local write "시"(w1362) -> ()
          }
        }
        "시간" <- w1300
        n817 = case shown="거짓" "초기화 2" {
          tunnel: [_ w1356] -> w1292
          tunnel: w1291 -> [_ w1351]
          tunnel: w1290 -> [_ w1357]
          frame False {
          }
          frame True {
            n818 = local read "Destination"() -> (w1353:string)
            n819 = local read "departure"() -> (w1354:string)
            n820 = Concatenate Strings(w1354, w1353, ":", w1351) -> (w1355:string)
            n821 = Build Array (concatenate)(w1355, w1357) -> (w1356:string[])
            n822 = global write "글로벌플라이트플랜.vi" "기록"(w1356) -> ()
          }
        }
      }
    }
  }
  n823 = invoke class="VI" method="FP.Close"(reference=w1) -> ()  [unwired: 2 in, 3 out]
